vi "musicplayer_next.vi"() -> ()   [LabVIEW 2012]
uses:
  System.Windows.Forms
  <vilib>/Utility/sysdir.llb/System Directory Type.ctl
  NotifyIcon/TypeDefs/NotifyIcon Events.ctl
  NotifyIcon/TypeDefs/NotifyIcon Event Registration Actions.ctl
  musicplayer_glo.vi
  <vilib>/Utility/cursorutil.llb/Set Cursor (Icon Pict).vi
  player_glo.vi
  debug_glo.vi
panel:
  out "ok_str":string
  in  "ok_but":bool
  in  "chase":dbl
  out "playwhile-brake":bool
  out "dataPfad":path
  out "NotifyIcon reference out":refnum<k24>
  out "pause?":bool=TRUE
  out "playlist referenz":refnum<vi>
  out "error-pool":errorcluster caption="Fehler (Ausgang)"
  out "playerkernel referenz":refnum<vi>
  out "version":string
  out "configPfad":path
  in  "ProgressBar":refnum<k24>(container)
  out "verdeckung":bool=TRUE
  in  "switch":bool
  in  "stop":bool
  in  "zufall":bool caption="random"
  out "playalone-titel":string caption="Einzeltitel:"
  in  "nachtitelpausieren":bool caption="last titel"
  in  "wiederholart":enum8{"False", "True", "Mixed"}(c332)
  in  "nechstentitel":bool
  in  "abspielen-einzeln":bool
  in  "pause":bool
  in  "play":bool
  in  "Volume":i64(slide) caption="Lautstärke" min=0 max=100 scale=0.1..100.0
  in  "balance":i8(slide) caption="Balance" scale=-10.0..10.0
  in  "position":ext(slide) caption="Position" scale=-1.0..1.0
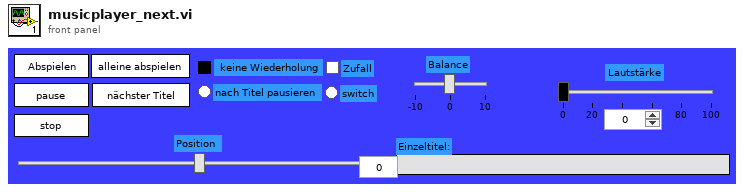
[diagram p1: front panel]
types:
  T1 = typedef "Window Refnum" = refnum<k1>
  T2 = enum32{"Invalid", "Standard", "Closed", "Hidden", "Minimized", "Maximized"}
  T3 = typedef "NotifyIcon Event Registration Actions.ctl" = enum16{"Initial Event Registration", "Add to Event Registration", "Destroy Events and Re-register"}
  T4 = enum8{"Enabled", "Disabled", "Disabled and Grayed Out"}
  T5 = typedef "System Directory Type.ctl" = i32
  T6 = typedef "NotifyIcon Events.ctl" = enum16{"BalloonTipClicked", "BalloonTipClosed", "BalloonTipShown", "Click", "Disposed", "DoubleClick", "MouseClick", "MouseDoubleClick", "MouseDown", "MouseMove", "MouseUp", "MenuItemClick", "MenuItemSelect"}
  T7 = typedef "NotifyIcon Event Data.ctl" = cluster{"NotifyIcon Event":T6, "Data String":string}
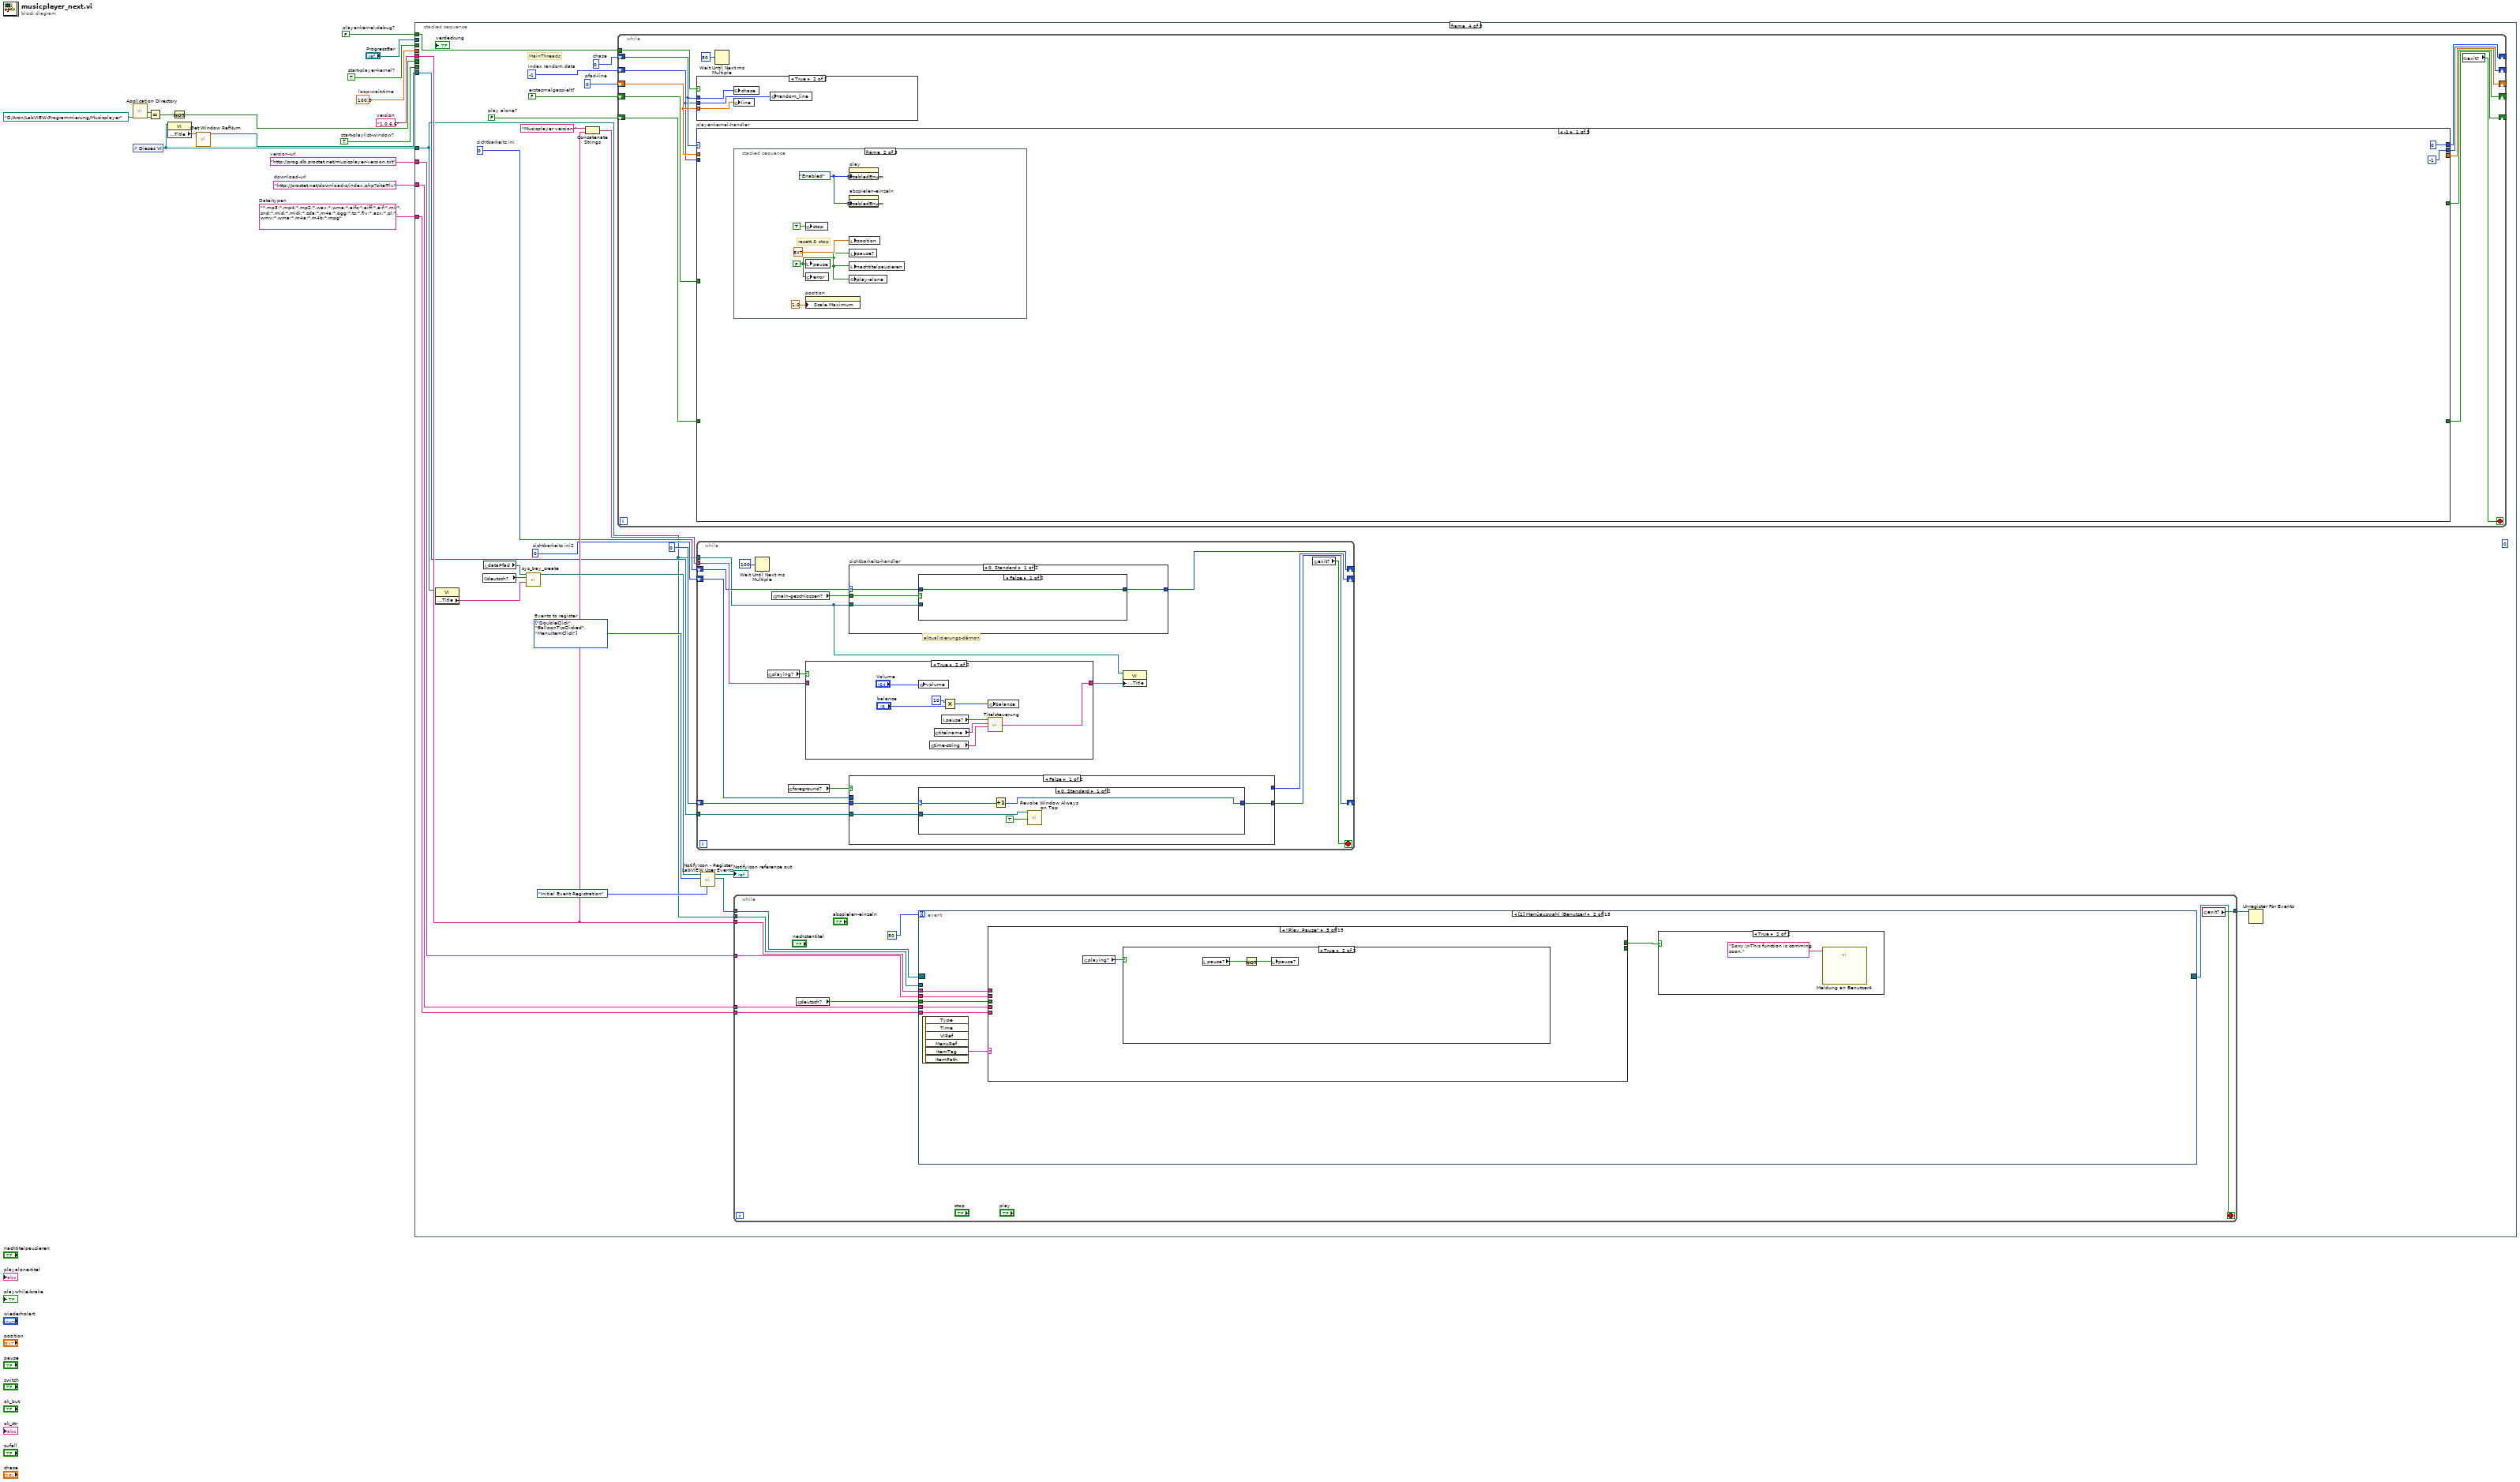
[diagram p0: block diagram]
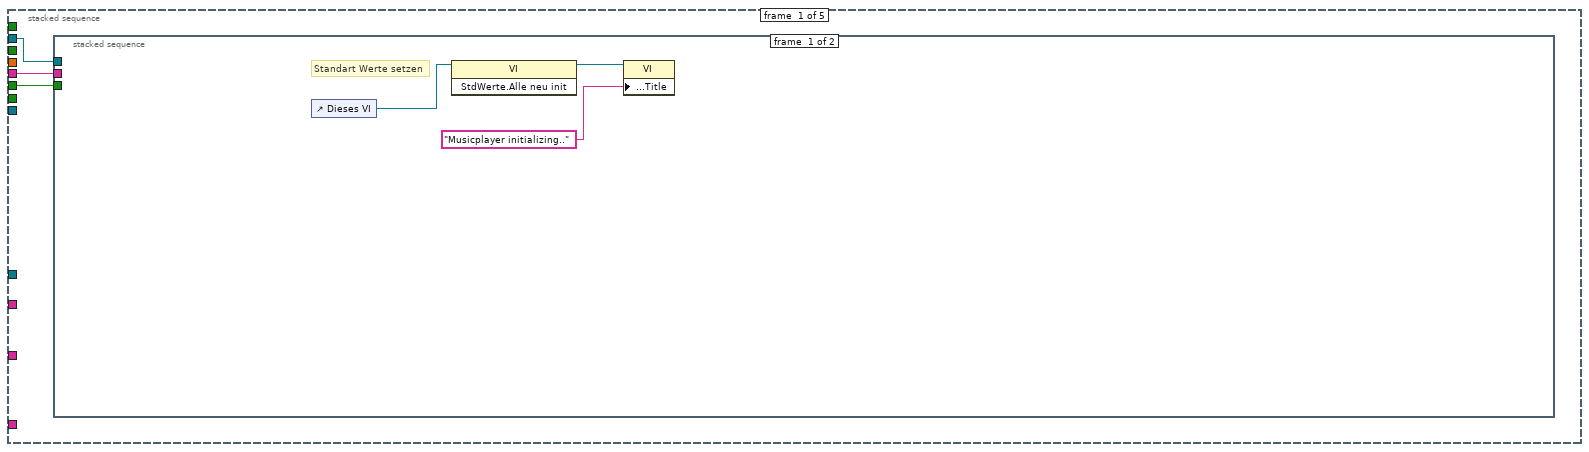
[diagram p2: hidden frame]
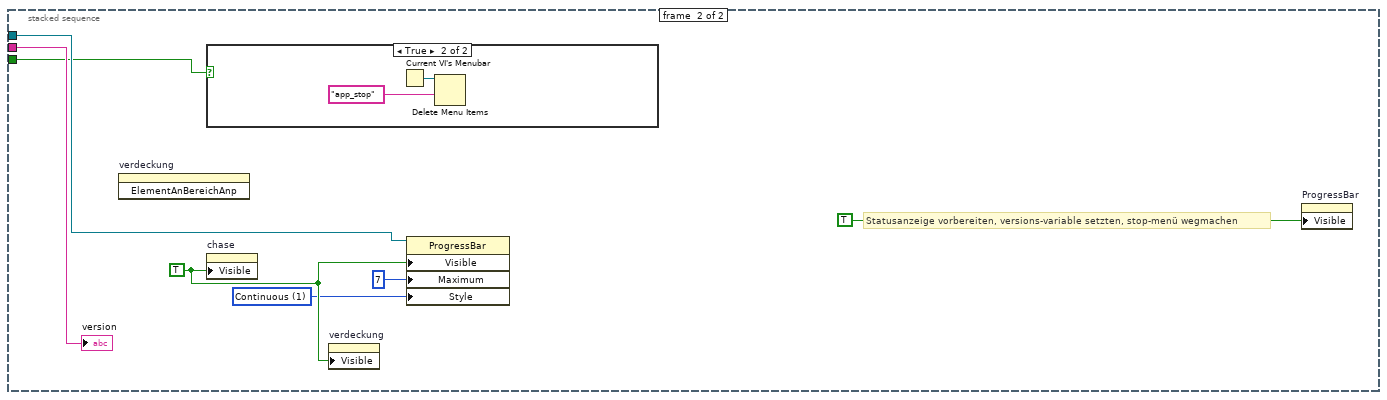
[diagram p3: hidden frame]
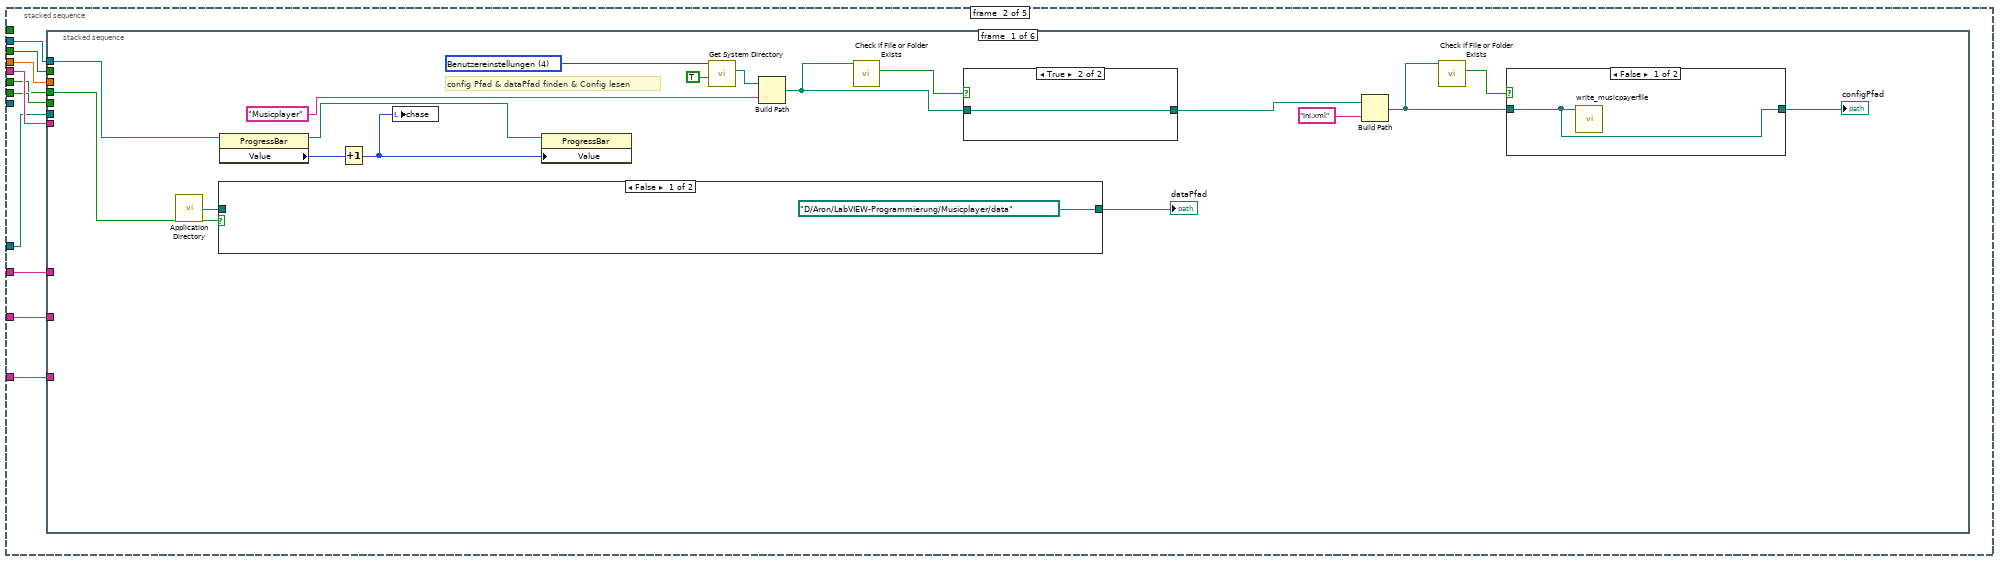
[diagram p5: hidden frame]
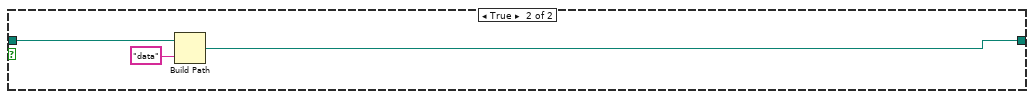
[diagram p6: hidden frame]
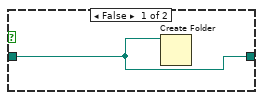
[diagram p8: hidden frame]
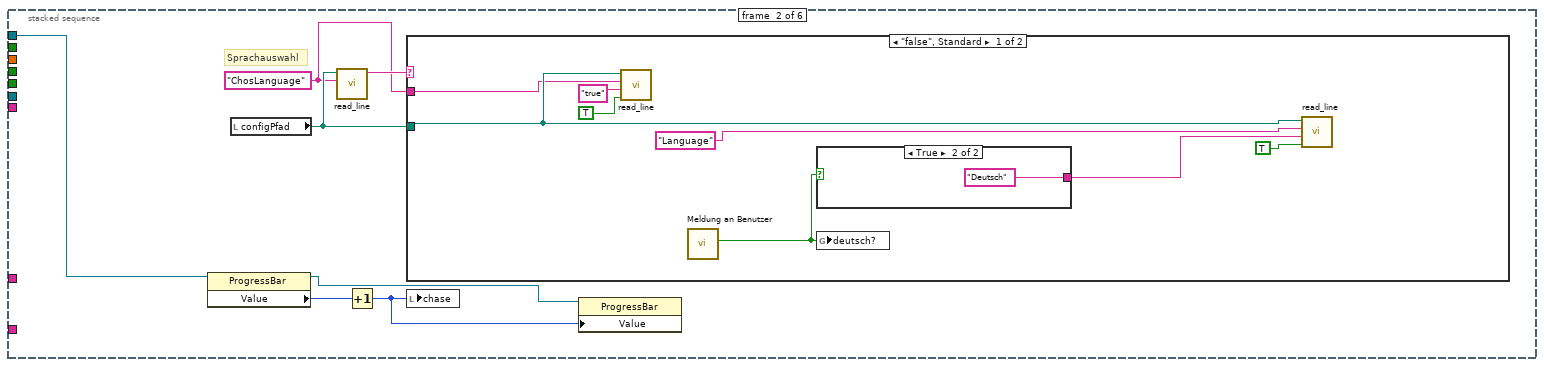
[diagram p9: hidden frame]
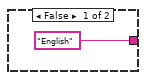
[diagram p10: hidden frame]
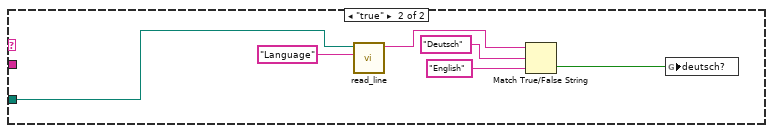
[diagram p11: hidden frame]
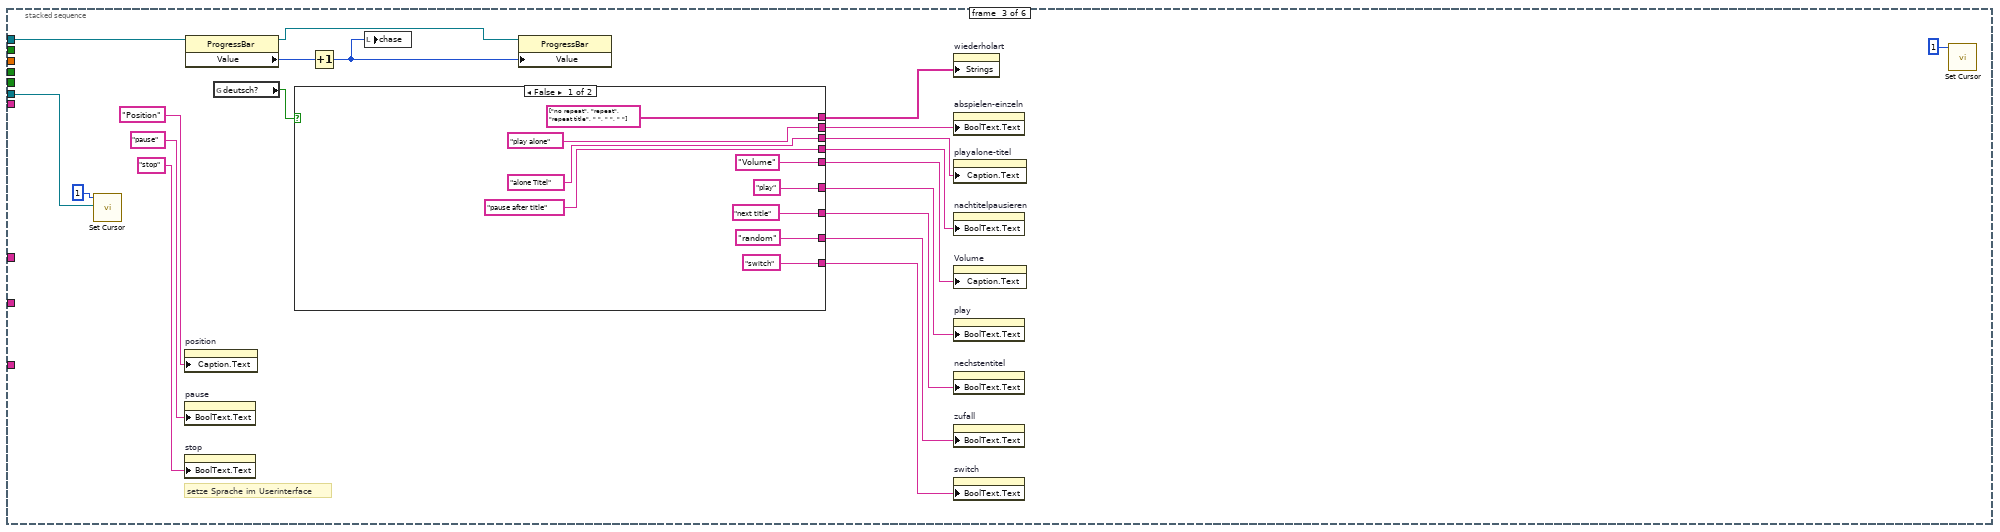
[diagram p12: hidden frame]
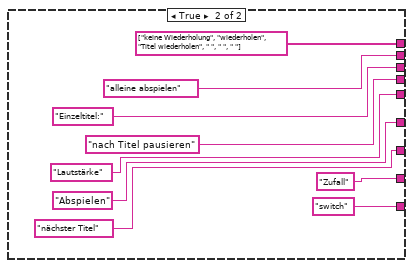
[diagram p13: hidden frame]
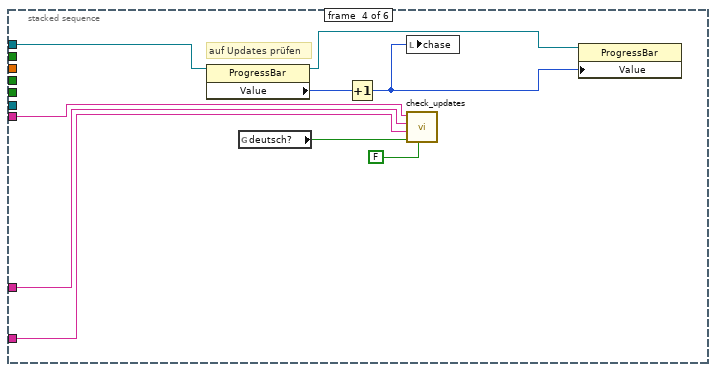
[diagram p14: hidden frame]
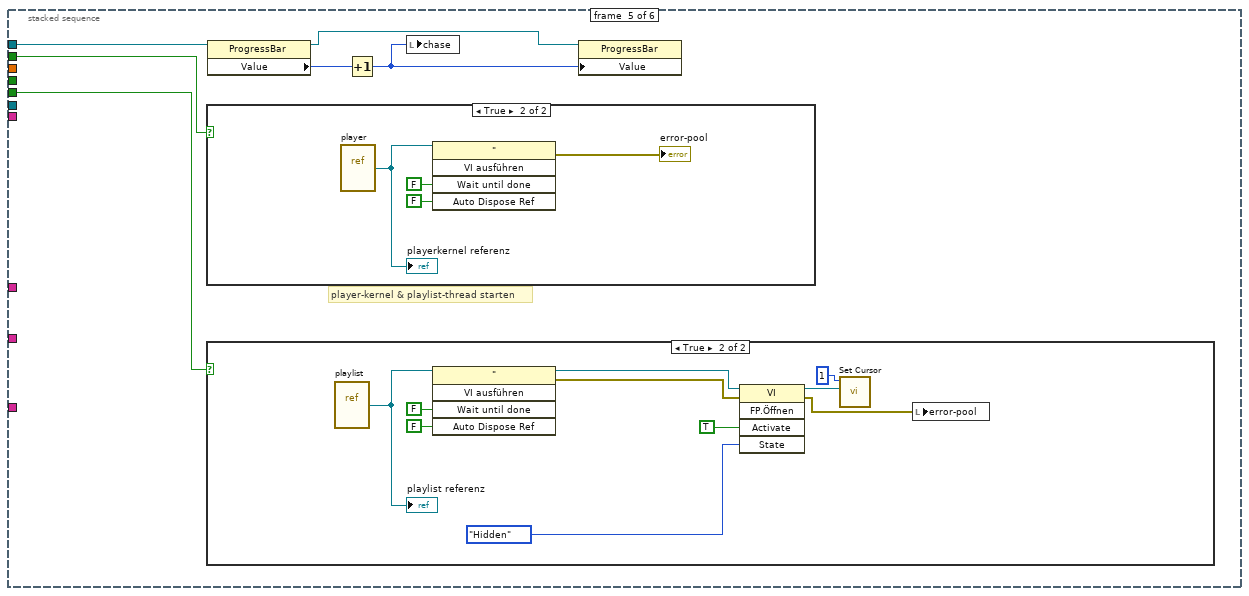
[diagram p15: hidden frame]
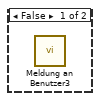
[diagram p16: hidden frame]
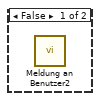
[diagram p17: hidden frame]
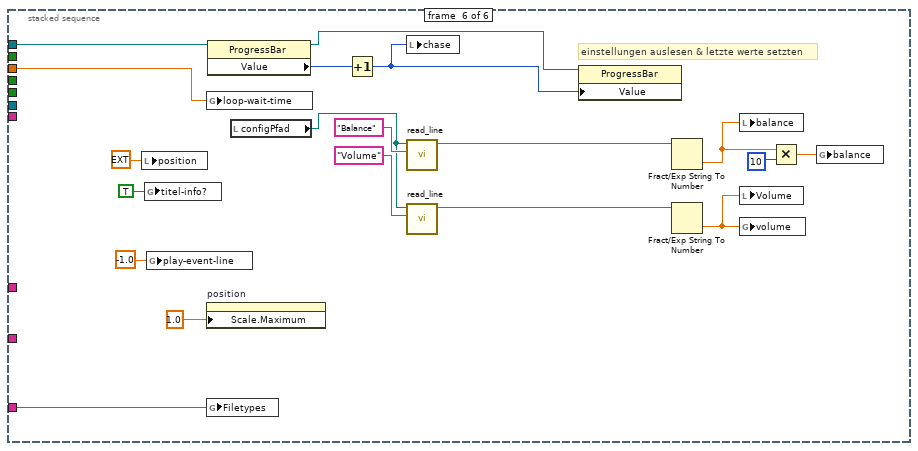
[diagram p18: hidden frame]
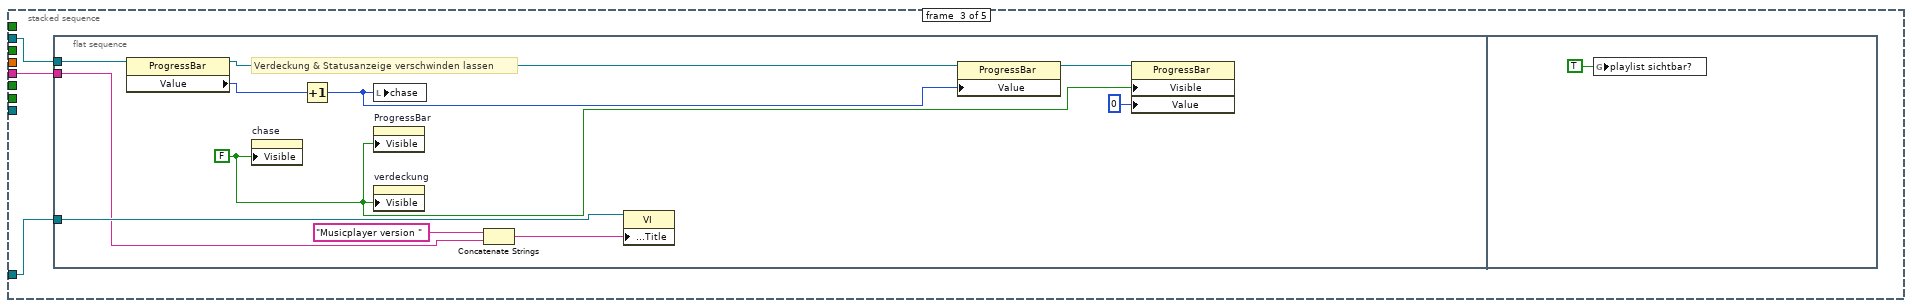
[diagram p19: hidden frame]
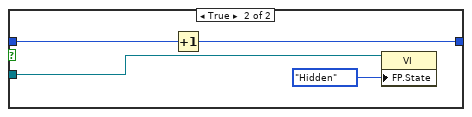
[diagram p20: hidden frame]
diagram:
  w1 = 100.0  # loop-wait-time
  w10 = "*.mp3;*.mp4;*.mp2;*.wav;*.wma;*.aifc;*.aiff;*.aif;*.mi;*.snd;*.mid;*.midi;*.cda;*.m4a;*.ogg;*.ts;*.flv;*.asx;*.pl;*.wmv;*.wma;*.m4a;*.m4b;*.mpg"  # Dateitypen
  w11 = FALSE  # player-kernel-debug?
  w12 = TRUE  # start-playlist-window?
  w13 = TRUE  # start-player-kernel?
  w14 = "http://proctet.net/download-s/index.php?site=lv"  # download-url
  w15 = "http://prog.db.proctet.net/musicplayer-version.txt"  # version-url
  w16 = "1.0.6.6"  # version
  n1 = call <vilib>:"Application Directory.vi"() -> ("Application Directory"=w6:path)
  n2 = control-ref of="Dieses VI"() -> (w4:refnum<vi>)
  n3 = Equal?(x=w6, y=path "D:/Aron/LabVIEW-Programmierung/Musicplayer" ("Zerlegter Pfad")) -> (x = y?=w8:bool)
  n4 = property class="VI"(reference=w4) -> ("Front Panel.Title"=w3:string)  [unwired: 1 in, 2 out]
  n5 = Not(x=w8) -> (.not. x?=w7:bool)
  n6 = call "Get Window RefNum.vi"("window name (\"\")"=w3) -> ("window refnum (NaWR)"=w2:T1)  [unwired: 7 in, 1 out]
  n7 = stacked-sequence {
    tunnel: "ProgressBar" -> [w19 w41 w177 _ _]
    tunnel: w16 -> [w18 w40 w178 w200 _]
    tunnel: w15 -> [_ w39 _ w198 _]
    tunnel: w14 -> [_ w38 _ w199 _]
    tunnel: w13 -> [_ w37 _ _ _]
    tunnel: w12 -> [_ w36 _ _ _]
    tunnel: w4 -> [_ w33 w179 w193 w857]
    tunnel: w11 -> [_ _ _ w212 _]
    tunnel: w10 -> [_ w35 _ w211 _]
    tunnel: w7 -> [w17 w34 _ _ _]
    tunnel: w2 -> [_ _ _ w196 _]
    tunnel: w1 -> [_ w32 _ _ _]
    frame #0 {
      n8 = stacked-sequence {
        tunnel: w19 -> [_ w28]
        tunnel: w18 -> [_ w26]
        tunnel: w17 -> [_ w25]
        frame #0 {
          # "Standart Werte setzen"
          n9 = control-ref of="Dieses VI"() -> (w22:refnum<vi>)
          n10 = invoke class="VI" method="StdWerte.Alle neu init"(reference=w22) -> (reference out=w21:refnum<vi>)  [unwired: 2 in, 2 out]
          n11 = property class="VI"(reference=w21, "Front Panel.Title"="Musicplayer initializing.." ("Frontpanel-Fenster:Titel")) -> ()  [unwired: 1 in, 2 out]
        }
        frame #1 {
          w23 = 1 items=["Blocks", "Continuous", "Marquee"] ("Style")
          w24 = TRUE ("Sichtbar")
          # "Statusanzeige vorbereiten, versions-variable setzten, stop-menü wegmachen"
          n12 = invoke on="verdeckung" class="Bool." method="ElementAnBereichAnp"() -> ()  [unwired: 3 in, 3 out]
          n13 = case shown="True" w25 {
            frame False {
            }
            frame True {
              n14 = Current VI's Menubar() -> (w31:refnum<k9>)
              n15 = Delete Menu Items(7:"app_stop" ("Objekte"), 9:w31) -> ()  [unwired: 2 in, 2 out]
            }
          }
          n16 = property on="chase" class="DigWert (strikt)"("Visible"=w24) -> ()  [unwired: 2 in, 2 out]
          n17 = property on="verdeckung" class="Bool."("Visible"=w24) -> ()  [unwired: 2 in, 2 out]
          n18 = property class="ProgressBar"(reference=w28, "Visible"=w24, "Maximum"=7, "Style"=w23) -> ()  [unwired: 1 in, 2 out]
          n19 = property on="ProgressBar" class="AXCont"("Visible"=TRUE ("Sichtbar")) -> ()  [unwired: 2 in, 2 out]
          "version" <- w26
        }
      }
    }
    frame #1 {
      n20 = stacked-sequence {
        tunnel: w41 -> [w48 w71 w108 w135 w141 w174]
        tunnel: w40 -> [_ _ _ w134 _ _]
        tunnel: w39 -> [_ _ _ w131 _ _]
        tunnel: w38 -> [_ _ _ w130 _ _]
        tunnel: w37 -> [_ _ _ _ w140 _]
        tunnel: w36 -> [_ _ _ _ w139 _]
        tunnel: w35 -> [_ _ _ _ _ w161]
        tunnel: w34 -> [w44 _ _ _ _ _]
        tunnel: w33 -> [_ _ w92 _ _ _]
        tunnel: w32 -> [_ _ _ _ _ w158]
        frame #0 {
          w59 = T5 4 items=["Benutzerverzeichnis"=0, "Benutzer-Desktop"=1, "Benutzerdokumente"=2, "Benutzeranwendungsdaten"=3, "Benutzereinstellungen"=4, "Temporäres Verzeichnis"=5, "Öffentliche Dokumente"=6, "Öffentliche Anwendungsdaten"=7, "Öffentliche Einstellungen"=8, "Öffentlicher Cache"=13, "Systembibliotheken"=9, "Installierte Bibliotheken"=10, "Applikationsdateien"=11, "Boot-Laufwerks-Stammverzeichnis"=12] ("system directory type")
          # "config Pfad & dataPfad finden & Config lesen"
          n21 = call <vilib>:"Application Directory.vi"() -> ("Application Directory"=w43:path)
          n22 = case shown="False" w44 {
            tunnel: w43 -> [_ w63]
            tunnel: [path "D:/Aron/LabVIEW-Programmierung/Musicplayer/data" ("stripped path") w61] -> w45
            frame False {
            }
            frame True {
              n23 = Build Path(base path=w63, name or relative path="data" ("Name oder relativer Pfad")) -> (appended path=w61:path)
            }
          }
          "dataPfad" <- w45
          n24 = property class="ProgressBar"(reference=w48) -> (reference out=w47:refnum<k24>, "Value"=w46:i32)  [unwired: 1 in, 1 out]
          n25 = Increment(x=w46) -> (x+1=w42:i32)
          n26 = local write "chase"(w42) -> ()
          n27 = property class="ProgressBar"(reference=w47, "Value"=w42) -> ()  [unwired: 1 in, 2 out]
          n28 = call <vilib>:"Get System Directory.vi"("create directory if not found? (F)"=TRUE, "system directory type"=w59) -> ("system directory"=w58:path)  [unwired: 9 in]
          n29 = Build Path(base path=w58, name or relative path="Musicplayer" ("Name oder relativer Pfad")) -> (appended path=w54:path)
          n30 = call <vilib>:"Check if File or Folder Exists.vi"("path"=w54) -> ("file or folder exists?"=w55:bool)  [unwired: 8 in, 2 out]
          n31 = case shown="True" w55 {
            tunnel: w54 -> [w66 w67]
            tunnel: [w66 w67] -> w53
            frame False {
              n32 = Create Folder(path (use dialog)=w66) -> ()  [unwired: 2 in, 3 out]
            }
            frame True {
            }
          }
          n33 = Build Path(base path=w53, name or relative path="ini.xml" ("Name oder relativer Pfad")) -> (appended path=w50:path)
          n34 = call <vilib>:"Check if File or Folder Exists.vi"("path"=w50) -> ("file or folder exists?"=w51:bool)  [unwired: 8 in, 2 out]
          n35 = case shown="False" w51 {
            tunnel: w50 -> [w64 w65]
            tunnel: [w64 w65] -> w49
            frame False {
              n36 = call "write_musicpayerfile.vi"("New XML File path"=w64) -> ()  [unwired: 10 in, 1 out]
            }
            frame True {
            }
          }
          "configPfad" <- w49
        }
        frame #1 {
          w68 = "ChosLanguage" ("Search objekt")
          # "Sprachauswahl"
          n37 = property class="ProgressBar"(reference=w71) -> (reference out=w73:refnum<k24>, "Value"=w72:i32)  [unwired: 1 in, 1 out]
          n38 = local read "configPfad"() -> (w70:path)
          n39 = call "read_line.vi"("Search objekt"=w68, "path to XML document"=w70) -> ("Value"=w74:string)  [unwired: 9 in]
          n40 = Increment(x=w72) -> (x+1=w69:i32)
          n41 = case shown="\"false\", Standard" w74 {
            tunnel: w70 -> [w78 w89]
            tunnel: w68 -> [w75 _]
            frame "false", Default {
              n42 = call "read_line.vi"("write"=TRUE, "Writedata"="true", "Search objekt"=w75, "path to XML document"=w78) -> ()  [unwired: 7 in, 1 out]
              n43 = call "Meldung an Benutzer"() -> ("German"=w82:bool)  [unwired: 10 in, 1 out]
              n44 = case shown="True" w82 {
                tunnel: ["English" "Deutsch"] -> w76
                frame False {
                }
                frame True {
                }
              }
              n45 = global write "musicplayer_glo.vi" "deutsch?"(w82) -> ()
              n46 = call "read_line.vi"("write"=TRUE, "Writedata"=w76, "Search objekt"="Language", "path to XML document"=w78) -> ()  [unwired: 7 in, 1 out]
            }
            frame "true" {
              n47 = call "read_line.vi"("Search objekt"="Language", "path to XML document"=w89) -> ("Value"=w88:string)  [unwired: 9 in]
              n48 = Match True/False String(2:"English" ("False-String"), 3:"Deutsch" ("True-String"), 4:w88) -> (0:w85:bool)  [unwired: 1 out]
              n49 = global write "musicplayer_glo.vi" "deutsch?"(w85) -> ()
            }
          }
          n50 = local write "chase"(w69) -> ()
          n51 = property class="ProgressBar"(reference=w73, "Value"=w69) -> ()  [unwired: 1 in, 2 out]
        }
        frame #2 {
          # "setze Sprache im Userinterface"
          n52 = call-poly <vilib>:"Set Cursor.vi"("VI reference (current VI)"=w92, "icon"=u16 1) -> ()  [unwired: 8 in, 2 out]
          n53 = property on="position" class="Schieber (strikt)"("Caption.Text"="Position") -> ()  [unwired: 2 in, 2 out]
          n54 = property on="pause" class="Bool. (strikt)"("BoolText.Text"="pause") -> ()  [unwired: 2 in, 2 out]
          n55 = property on="stop" class="Bool."("BoolText.Text"="stop") -> ()  [unwired: 2 in, 2 out]
          n56 = property class="ProgressBar"(reference=w108) -> (reference out=w110:refnum<k24>, "Value"=w109:i32)  [unwired: 1 in, 1 out]
          n57 = global read "musicplayer_glo.vi" "deutsch?"() -> (w107:bool)
          n58 = case shown="False" w107 {
            tunnel: [string[] ["no repeat", "repeat", "repeat title", " ", " ", " "] string[] ["keine Wiederholung", "wiederholen", "Titel wiederholen", " ", " ", " "]] -> w100
            tunnel: ["play" "Abspielen"] -> w106
            tunnel: ["play alone" "alleine abspielen"] -> w105
            tunnel: ["next title" "nächster Titel"] -> w103
            tunnel: ["pause after title" "nach Titel pausieren"] -> w101
            tunnel: ["random" "Zufall"] -> w99
            tunnel: ["switch" "switch"] -> w98
            tunnel: ["Volume" "Lautstärke"] -> w97
            tunnel: ["alone Titel" "Einzeltitel:"] -> w95
            frame False {
            }
            frame True {
            }
          }
          n59 = Increment(x=w109) -> (x+1=w94:i32)
          n60 = local write "chase"(w94) -> ()
          n61 = property class="ProgressBar"(reference=w110, "Value"=w94) -> ()  [unwired: 1 in, 2 out]
          n62 = property on="wiederholart" class="3ZustandsFeld (strikt)"("Strings"=w100) -> ()  [unwired: 2 in, 2 out]
          n63 = property on="abspielen-einzeln" class="Bool."("BoolText.Text"=w105) -> ()  [unwired: 2 in, 2 out]
          n64 = property on="playalone-titel" class="Str"("Caption.Text"=w95) -> ()  [unwired: 2 in, 2 out]
          n65 = property on="nachtitelpausieren" class="Bool. (strikt)"("BoolText.Text"=w101) -> ()  [unwired: 2 in, 2 out]
          n66 = property on="Volume" class="Schieber (strikt)"("Caption.Text"=w97) -> ()  [unwired: 2 in, 2 out]
          n67 = property on="play" class="Bool."("BoolText.Text"=w106) -> ()  [unwired: 2 in, 2 out]
          n68 = property on="nechstentitel" class="Bool."("BoolText.Text"=w103) -> ()  [unwired: 2 in, 2 out]
          n69 = property on="zufall" class="Bool. (strikt)"("BoolText.Text"=w99) -> ()  [unwired: 2 in, 2 out]
          n70 = property on="switch" class="Bool. (strikt)"("BoolText.Text"=w98) -> ()  [unwired: 2 in, 2 out]
          n71 = call-poly <vilib>:"Set Cursor.vi"("icon"=u16 1) -> ()  [unwired: 9 in, 2 out]
        }
        frame #3 {
          # "auf Updates prüfen"
          n72 = property class="ProgressBar"(reference=w135) -> (reference out=w137:refnum<k24>, "Value"=w136:i32)  [unwired: 1 in, 1 out]
          n73 = global read "musicplayer_glo.vi" "deutsch?"() -> (w133:bool)
          n74 = Increment(x=w136) -> (x+1=w129:i32)
          n75 = local write "chase"(w129) -> ()
          n76 = call "check_updates.vi"("dialog by newest version?"=FALSE, "german?"=w133, "downloadpath"=w130, "get-path"=w131, "current version"=w134) -> ()  [unwired: 6 in, 1 out]
          n77 = property class="ProgressBar"(reference=w137, "Value"=w129) -> ()  [unwired: 1 in, 2 out]
        }
        frame #4 {
          # "player-kernel & playlist-thread starten"
          n78 = case shown="True" w140 {
            frame False {
              n79 = call "Meldung an Benutzer2"() -> ()  [unwired: 10 in, 2 out]
            }
            frame True {
              n80 = vi-ref "player.vi"() -> (w155:refnum<vi>)
              "playerkernel referenz" <- w155
              n81 = invoke class="\"" method="VI ausführen"(reference=w155, "Wait until done"=FALSE ("Warten bis beendet"), "Auto Dispose Ref"=FALSE ("Referenz automatisch schließen")) -> (error out=→"error-pool":errorcluster)  [unwired: 2 in, 4 out]
            }
          }
          n82 = case shown="True" w139 {
            frame False {
              n83 = call "Meldung an Benutzer3"() -> ()  [unwired: 10 in, 2 out]
            }
            frame True {
              n84 = vi-ref "playlist.vi"() -> (w151:refnum<vi>)
              "playlist referenz" <- w151
              n85 = invoke class="\"" method="VI ausführen"(reference=w151, "Wait until done"=FALSE ("Warten bis beendet"), "Auto Dispose Ref"=FALSE ("Referenz automatisch schließen")) -> (reference out=w150:refnum<vi>, error out=w149:errorcluster)  [unwired: 2 in, 3 out]
              n86 = invoke class="VI" method="FP.Öffnen"(reference=w150, error in=w149, "Activate"=TRUE ("Aktivieren?"), "State"=T2."Hidden" ("Zustand")) -> (reference out=w144:refnum<vi>, error out=w148:errorcluster)  [unwired: 1 in, 3 out]
              n87 = call-poly <vilib>:"Set Cursor.vi"("VI reference (current VI)"=w144, "icon"=u16 1) -> ()  [unwired: 8 in, 2 out]
              n88 = local write "error-pool"(w148) -> ()
            }
          }
          n89 = property class="ProgressBar"(reference=w141) -> (reference out=w143:refnum<k24>, "Value"=w142:i32)  [unwired: 1 in, 1 out]
          n90 = Increment(x=w142) -> (x+1=w138:i32)
          n91 = local write "chase"(w138) -> ()
          n92 = property class="ProgressBar"(reference=w143, "Value"=w138) -> ()  [unwired: 1 in, 2 out]
        }
        frame #5 {
          # "einstellungen auslesen & letzte werte setzten"
          n93 = local write "position"(ext 1.0 ("position")) -> ()
          n94 = global write "musicplayer_glo.vi" "titel-info?"(TRUE ("titel-info?")) -> ()
          n95 = global write "musicplayer_glo.vi" "play-event-line"(-1.0 ("play-event-line")) -> ()
          n96 = global write "player_glo.vi" "loop-wait-time"(w158) -> ()
          n97 = property on="position" class="Schieber (strikt)"("Scale.Maximum"=1.0 ("Skalierung.Bereich:Maximum")) -> ()  [unwired: 2 in, 2 out]
          n98 = global write "musicplayer_glo.vi" "Filetypes"(w161) -> ()
          n99 = property class="ProgressBar"(reference=w174) -> (reference out=w176:refnum<k24>, "Value"=w175:i32)  [unwired: 1 in, 1 out]
          n100 = local read "configPfad"() -> (w167:path)
          n101 = Increment(x=w175) -> (x+1=w159:i32)
          n102 = local write "chase"(w159) -> ()
          n103 = call "read_line.vi"("Search objekt"="Balance", "path to XML document"=w167) -> ("Value"=w172:string)  [unwired: 9 in]
          n104 = call "read_line.vi"("Search objekt"="Volume", "path to XML document"=w167) -> ("Value"=w168:string)  [unwired: 9 in]
          n105 = property class="ProgressBar"(reference=w176, "Value"=w159) -> ()  [unwired: 1 in, 2 out]
          n106 = Fract/Exp String To Number(string=w172) -> (number=w165:dbl)  [unwired: 4 out]
          n107 = Fract/Exp String To Number(string=w168) -> (number=w166:dbl)  [unwired: 4 out]
          n108 = local write "balance"(w165) -> ()
          n109 = local write "Volume"(w166) -> ()
          n110 = global write "player_glo.vi" "volume"(w166) -> ()
          n111 = Multiply(x=w165, y=10 ("Offset nach Zahl")) -> (x*y=w170:dbl)
          n112 = global write "player_glo.vi" "balance"(w170) -> ()
        }
      }
    }
    frame #2 {
      n113 = flat-sequence {
        tunnel: w179 -> [w189]
        tunnel: w178 -> [w186]
        tunnel: w177 -> [w183]
        frame #0 {
          w180 = FALSE ("Visible")
          # "Verdeckung & Statusanzeige verschwinden lassen"
          n114 = property class="ProgressBar"(reference=w183) -> (reference out=w185:refnum<k24>, "Value"=w184:i32)  [unwired: 1 in, 1 out]
          n115 = property on="chase" class="DigWert (strikt)"("Visible"=w180) -> ()  [unwired: 2 in, 2 out]
          n116 = Increment(x=w184) -> (x+1=w181:i32)
          n117 = local write "chase"(w181) -> ()
          n118 = property on="ProgressBar" class="AXCont"("Visible"=w180) -> ()  [unwired: 2 in, 2 out]
          n119 = property on="verdeckung" class="Bool."("Visible"=w180) -> ()  [unwired: 2 in, 2 out]
          n120 = Concatenate Strings("Musicplayer version " ("String"), w186) -> (w188:string)
          n121 = property class="VI"(reference=w189, "Front Panel.Title"=w188) -> ()  [unwired: 1 in, 2 out]
          n122 = property class="ProgressBar"(reference=w185, "Value"=w181) -> (reference out=w182:refnum<k24>)  [unwired: 1 in, 1 out]
          n123 = property class="ProgressBar"(reference=w182, "Visible"=w180, "Value"=0) -> ()  [unwired: 1 in, 2 out]
        }
        frame #1 {
          n124 = global write "musicplayer_glo.vi" "playlist sichtbar?"(TRUE ("playlist sichtbar?")) -> ()
        }
      }
    }
    frame #3 {
      w195 = 0  # sichtbarkeits ini2
      w197 = 0  # sichtbarkeits ini
      w206 = T6[] [enum."DoubleClick", enum."BalloonTipClicked", enum."MenuItemClick"] items=["BalloonTipClicked", "BalloonTipClosed", "BalloonTipShown", "Click", "Disposed", "DoubleClick", "MouseClick", "MouseDoubleClick", "MouseDown", "MouseMove", "MouseUp", "MenuItemClick", "MenuItemSelect"]  # Events to register
      (unwired) 0
      w213 = -1  # index random data
      w214 = FALSE  # play alone?
      w215 = 0  # pfad-line
      w216 = FALSE  # erstesmalgespielt?
      w217 = 0  # chase
      # "MainThreads"
      n125 = property class="VI"(reference=w193) -> ("Front Panel.Title"=w192:string)  [unwired: 1 in, 2 out]
      n126 = global read "musicplayer_glo.vi" "deutsch?"() -> (w203:bool)
      n127 = local read "dataPfad"() -> (w201:path)
      n128 = call "sys_tray_create.vi"("hover-text"=w192, "deutsch?"=w203, "data_pfad"=w201) -> ("NotifyIcon reference out"=w207:refnum<k24>)  [unwired: 8 in]
      n129 = Concatenate Strings("Musicplayer version " ("String"), w200) -> (w209:string)
      n130 = while {
        shift-right: [w495] -> _
        shift-left: w217 -> [w486]
        shift-right: [w494] -> _
        shift-left: w215 -> [w485]
        shift-right: [w493] -> _
        shift-left: w214 -> [w492]
        shift-right: [w490] -> _
        shift-left: w216 -> [w491]
        shift-right: [w489] -> _
        shift-left: w213 -> [w484]
        tunnel: w212 -> [w488]
        stop <- w487 stop-if-true
        n131 = case shown="True" w488 {
          tunnel: w486 -> [_ w499]
          tunnel: w485 -> [_ w498]
          tunnel: w484 -> [_ w497]
          frame False {
          }
          frame True {
            n132 = global write "debug_glo.vi" "chase"(w499) -> ()
            n133 = global write "debug_glo.vi" "line"(w498) -> ()
            n134 = global write "debug_glo.vi" "random_line"(w497) -> ()
          }
        }
        n135 = case "player-kernel-handler" shown="-1" w486 {
          selector: w486 -> [_ w511 w530 _ _]
          tunnel: [0 w510 w528 w729 w772] -> w495
          tunnel: [_ -1 w525 w733 w773] -> w494
          tunnel: w485 -> [_ _ w526 w733 w773]
          tunnel: [_ _ w531 w732 w769] -> w493
          tunnel: w492 -> [_ _ _ w732 w769]
          tunnel: w491 -> [_ _ w527 w731 _]
          tunnel: [_ _ _ w731 w770] -> w490
          tunnel: w484 -> [_ _ w524 w730 w771]
          tunnel: [-1 -1 w522 w730 w771] -> w489
          frame -1 {
            n136 = stacked-sequence {
              frame #0 {
                n137 = global write "musicplayer_glo.vi" "stop-event"(TRUE ("stop-event")) -> ()
              }
              frame #1 {
                w507 = T4."Enabled" ("Deaktiviert")
                w504 = FALSE ("play-alone")
                # "resett & stop"
                n138 = global write "player_glo.vi" "stop"(TRUE ("stop")) -> ()
                n139 = local write "pause"(w504) -> ()
                n140 = global write "player_glo.vi" "error"(w504) -> ()
                n141 = property on="position" class="Schieber (strikt)"("Scale.Maximum"=1.0 ("Skalierung.Bereich:Maximum")) -> ()  [unwired: 2 in, 2 out]
                n142 = property on="play" class="Bool."("DisabledEnum"=w507) -> ()  [unwired: 2 in, 2 out]
                n143 = property on="abspielen-einzeln" class="Bool."("DisabledEnum"=w507) -> ()  [unwired: 2 in, 2 out]
                n144 = local write "position"(ext 0.0 ("position")) -> ()
                n145 = local write "pause?"(w504) -> ()
                n146 = local write "nachtitelpausieren"(w504) -> ()
                n147 = global write "musicplayer_glo.vi" "play-alone"(w504) -> ()
              }
              frame #2 {
                n148 = global write "musicplayer_glo.vi" "stop-event"(FALSE ("stop-event")) -> ()
              }
            }
          }
          frame 0, Default {
            n149 = global read "musicplayer_glo.vi" "play-event"() -> (w512:bool)
            n150 = case "play-event-handler" shown="True" w512 {
              tunnel: w511 -> [w514 _]
              tunnel: [w514 1] -> w510
              frame False {
              }
              frame True {
              }
            }
          }
          frame 1 {
            w518 = FALSE ("stop-event")
            w521 = T4."Disabled and Grayed Out" ("Deaktiviert")
            n151 = global read "musicplayer_glo.vi" "play-alone"() -> (w531:bool)
            n152 = global read "musicplayer_glo.vi" "play-event"() -> (w534:bool)
            n153 = local write "pause"(w518) -> ()
            n154 = local read "nachtitelpausieren"() -> (w517:bool)
            n155 = global read "musicplayer_glo.vi" "play-event-line"() -> (w532:dbl)
            n156 = global write "musicplayer_glo.vi" "stop-event"(w518) -> ()
            n157 = local write "playwhile-brake"(w518) -> ()
            n158 = local write "pause?"(w518) -> ()
            n159 = case shown="True" w517 {
              frame False {
              }
              frame True {
                n160 = property on="nachtitelpausieren" class="Bool. (strikt)"("DisabledEnum"=T4."Disabled and Grayed Out" ("Deaktiviert")) -> ()  [unwired: 2 in, 2 out]
              }
            }
            n161 = local read "switch"() -> (w519:bool)
            n162 = local read "zufall"() -> (w523:bool)
            n163 = property on="play" class="Bool."("DisabledEnum"=w521) -> ()  [unwired: 2 in, 2 out]
            n164 = property on="abspielen-einzeln" class="Bool."("DisabledEnum"=w521) -> ()  [unwired: 2 in, 2 out]
            n165 = case "play-event?" shown="False" w534 {
              tunnel: w531 -> [w548 w703]
              tunnel: w532 -> [_ w697]
              tunnel: [w547 w702] -> w533
              tunnel: [w546 _] -> w529
              tunnel: w527 -> [w545 _]
              tunnel: w526 -> [w544 _]
              tunnel: [w543 w701] -> w525
              tunnel: w524 -> [w541 w700]
              tunnel: w523 -> [w542 w699]
              tunnel: [w540 w698] -> w522
              tunnel: [_ FALSE ("play-event")] -> w520
              tunnel: w519 -> [w539 _]
              frame False {
                n166 = case "switch?" shown="False" w539 {
                  tunnel: w548 -> [w557 w663]
                  tunnel: [w556 w658] -> w547
                  tunnel: [w555 w661] -> w546
                  tunnel: w545 -> [w554 _]
                  tunnel: w544 -> [w553 _]
                  tunnel: [w549 w659] -> w543
                  tunnel: w542 -> [w552 w662]
                  tunnel: w541 -> [w551 _]
                  tunnel: [w550 w660] -> w540
                  frame False {
                    n167 = local read "wiederholart"() -> (w558:enum8{"False", "True", "Mixed"})
                    n168 = case "play-alone?" shown="False" w557 {
                      tunnel: w558 -> [w565 w648]
                      tunnel: [w562 w647] -> w556
                      tunnel: [w561 w646] -> w555
                      tunnel: w554 -> [_ w645]
                      tunnel: w553 -> [w566 w643]
                      tunnel: w552 -> [w563 _]
                      tunnel: w551 -> [w564 _]
                      tunnel: [w559 -1] -> w550
                      tunnel: [w560 w643] -> w549
                      frame False {
                        n169 = case "zufall?" shown="False" w563 {
                          tunnel: w565 -> [w568 w602]
                          tunnel: [w572 w599] -> w562
                          tunnel: [w571 w601] -> w561
                          tunnel: [w570 w595] -> w560
                          tunnel: w564 -> [_ w597]
                          tunnel: [-1 w600] -> w559
                          tunnel: w566 -> [w567 _]
                          frame False {
                            n170 = global read "musicplayer_glo.vi" "pfade"() -> (w577:string[])
                            n171 = Array Size(array=w577) -> (size(s)=w576:i32)
                            n172 = Subtract(x=w576, y=1 ("Größe(n)")) -> (x-y=w574:i32)
                            n173 = Equal?(x=w567, y=w574) -> (x = y?=w573:bool)
                            n174 = case "lezter titel?" shown="True" w573 {
                              tunnel: w568 -> [w579 w591]
                              tunnel: [w581 w589] -> w572
                              tunnel: [_ w592] -> w571
                              tunnel: [w580 w588] -> w570
                              tunnel: w567 -> [w578 _]
                              frame False {
                                n175 = Equal?(x=w579, y=enum8{"False", "True", "Mixed"}."Mixed") -> (x = y?=w582:bool)
                                n176 = case "titel wiederholen?" shown="False" w582 {
                                tunnel: [w586 w587] -> w580
                                tunnel: w578 -> [w585 w587]
                                frame False {
                                n177 = Increment(x=w585) -> (x+1=w586:ext)
                                }
                                frame True {
                                }
                                }
                                n178 = global read "musicplayer_glo.vi" "pfade"() -> (w583:string[])
                                n179 = Index Array(array=w583, index=w580) -> (element=w581:string)
                              }
                              frame True {
                                n180 = case "wiederholart" shown="\"False\", Standard" w591 {
                                tunnel: [TRUE _ _] -> w592
                                tunnel: [_ 0 _] -> w588
                                frame "False", Default {
                                }
                                frame "True" {
                                }
                                frame "Mixed" {
                                }
                                }
                                n181 = global read "musicplayer_glo.vi" "pfade"() -> (w590:string[])
                                n182 = Index Array(array=w590, index=w588) -> (element=w589:string)
                              }
                            }
                          }
                          frame True {
                            n183 = Not Equal?(x=w597, y=-1) -> (x != y?=w596:bool)
                            n184 = case "zufallswerte generiert?" shown="False" w596 {
                              tunnel: w602 -> [_ w618]
                              tunnel: [_ w617] -> w601
                              tunnel: [w605 w616] -> w600
                              tunnel: w597 -> [_ w614]
                              tunnel: [w604 w615] -> w599
                              tunnel: [w603 w612] -> w595
                              frame False {
                                n185 = stacked-sequence {
                                tunnel: [_ w609] -> w605
                                tunnel: [_ w608] -> w604
                                tunnel: [_ w606] -> w603
                                frame #0 {
                                n186 = call "write_random_data.vi"() -> ()  [unwired: 12 in]
                                }
                                frame #1 {
                                w609 = 0
                                n187 = global read "musicplayer_glo.vi" "random-data"() -> (w607:ext[])
                                n188 = Index Array(array=w607, index=w609) -> (element=w606:ext)
                                n189 = global read "musicplayer_glo.vi" "pfade"() -> (w610:string[])
                                n190 = Index Array(array=w610, index=w606) -> (element=w608:string)
                                }
                                }
                              }
                              frame True {
                                n191 = global read "musicplayer_glo.vi" "random-data"() -> (w611:ext[])
                                n192 = Array Size(array=w611) -> (size(s)=w613:i32)
                                n193 = Greater Or Equal?(x=w614, y=w613) -> (x >= y?=w619:bool)
                                n194 = case "lezter zufallswert?" shown="True" w619 {
                                tunnel: w618 -> [w624 w639]
                                tunnel: [_ w638] -> w617
                                tunnel: [w622 w634] -> w616
                                tunnel: w614 -> [w623 w637]
                                tunnel: [w627 w635] -> w615
                                tunnel: w611 -> [w621 w633]
                                tunnel: [w620 w632] -> w612
                                frame False {
                                n195 = Equal?(x=w624, y=enum8{"False", "True", "Mixed"}."Mixed") -> (x = y?=w625:bool)
                                n196 = case "titel wiederholen?" shown="True" w625 {
                                tunnel: w623 -> [w629 w631]
                                tunnel: [w630 w631] -> w622
                                frame False {
                                n197 = Increment(x=w629) -> (x+1=w630:i32)
                                }
                                frame True {
                                }
                                }
                                n198 = Index Array(array=w621, index=w622) -> (element=w620:ext)
                                n199 = global read "musicplayer_glo.vi" "pfade"() -> (w628:string[])
                                n200 = Index Array(array=w628, index=w620) -> (element=w627:string)
                                }
                                frame True {
                                n201 = case "wiederholung?" shown="\"Mixed\"" w639 {
                                tunnel: [TRUE _ _] -> w638
                                tunnel: [_ 0 w642] -> w634
                                tunnel: w637 -> [_ _ w642]
                                frame "False", Default {
                                }
                                frame "True" {
                                }
                                frame "Mixed" {
                                }
                                }
                                n202 = Index Array(array=w633, index=w634) -> (element=w632:ext)
                                n203 = global read "musicplayer_glo.vi" "pfade"() -> (w636:string[])
                                n204 = Index Array(array=w636, index=w632) -> (element=w635:string)
                                }
                                }
                              }
                            }
                          }
                        }
                      }
                      frame True {
                        n205 = case "wiederholgung?" shown="\"False\", Standard" w648 {
                          tunnel: [w649 w654 w655] -> w647
                          tunnel: [w651 _ _] -> w646
                          tunnel: w645 -> [w650 _ _]
                          frame "False", Default {
                            n206 = case "schonmal gespielt?" shown="True" w650 {
                              tunnel: [_ TRUE] -> w651
                              tunnel: [w652 _] -> w649
                              frame False {
                                n207 = global read "musicplayer_glo.vi" "playlone-lied-Pfad"() -> (w652:string)
                              }
                              frame True {
                              }
                            }
                          }
                          frame "True" {
                            n208 = global read "musicplayer_glo.vi" "playlone-lied-Pfad"() -> (w654:string)
                          }
                          frame "Mixed" {
                            n209 = global read "musicplayer_glo.vi" "playlone-lied-Pfad"() -> (w655:string)
                          }
                        }
                      }
                    }
                  }
                  frame True {
                    n210 = case "play-alone?" shown="True" w663 {
                      tunnel: w662 -> [_ w677]
                      tunnel: [_ w672] -> w661
                      tunnel: [-1 w671] -> w660
                      tunnel: [_ w669] -> w659
                      tunnel: [w665 w668] -> w658
                      tunnel: [TRUE FALSE] -> w657
                      frame False {
                        n211 = global read "musicplayer_glo.vi" "playlone-lied-Pfad"() -> (w665:string)
                      }
                      frame True {
                        n212 = global read "musicplayer_glo.vi" "pfade"() -> (w675:string[])
                        n213 = Index Array(array=w675, index=0 ("Index")) -> (element=w670:string)
                        n214 = Not Equal?(x=w670, y="") -> (x != y?=w673:bool)
                        n215 = case "leere playlist?" shown="True" w673 {
                          tunnel: w677 -> [_ w684]
                          tunnel: [TRUE _] -> w672
                          tunnel: [-1 w682] -> w671
                          tunnel: w670 -> [_ w683]
                          tunnel: [_ w681] -> w669
                          tunnel: [_ w680] -> w668
                          frame False {
                          }
                          frame True {
                            n216 = case "zufall?" shown="True" w684 {
                              tunnel: w683 -> [w685 _]
                              tunnel: [-1 w690] -> w682
                              tunnel: [0 w688] -> w681
                              tunnel: [w685 w689] -> w680
                              frame False {
                              }
                              frame True {
                                n217 = stacked-sequence {
                                tunnel: [_ w693] -> _
                                tunnel: [_ w694] -> w689
                                tunnel: [_ w693] -> w690
                                tunnel: [_ w691] -> w688
                                frame #0 {
                                n218 = call "write_random_data.vi"() -> ()  [unwired: 12 in]
                                }
                                frame #1 {
                                w693 = 0
                                n219 = global read "musicplayer_glo.vi" "random-data"() -> (w692:ext[])
                                n220 = Index Array(array=w692, index=w693) -> (element=w691:ext)
                                n221 = global read "musicplayer_glo.vi" "pfade"() -> (w695:string[])
                                n222 = Index Array(array=w695, index=w691) -> (element=w694:string)
                                }
                                }
                              }
                            }
                          }
                        }
                      }
                    }
                    n223 = local write "switch"(FALSE ("switch")) -> ()
                    n224 = global write "musicplayer_glo.vi" "play-alone"(w657) -> ()
                  }
                }
              }
              frame True {
                n225 = case "play alone?" shown="False" w703 {
                  tunnel: [w713 w728] -> w702
                  tunnel: [w711 _] -> w701
                  tunnel: w700 -> [w712 _]
                  tunnel: w699 -> [w710 _]
                  tunnel: [w709 -1] -> w698
                  tunnel: w697 -> [w704 _]
                  frame False {
                    n226 = Not Equal?(x=w704, y=-1.0) -> (x != y?=w705:bool)
                    n227 = Not(x=w705) -> (.not. x?=w706:bool)
                    n228 = And(x=w710, y=w706) -> (x .and. y?=w707:bool)
                    n229 = case "zufall, & kein line-festgelegt?" shown="True" w707 {
                      tunnel: w712 -> [_ w723]
                      tunnel: w704 -> [w717 _]
                      tunnel: [w718 w721] -> w711
                      tunnel: [-1 w722] -> w709
                      tunnel: w705 -> [w716 _]
                      frame False {
                        n230 = case shown="False" w716 {
                          tunnel: [0 w720] -> w718
                          tunnel: w717 -> [_ w720]
                          frame False {
                          }
                          frame True {
                          }
                        }
                      }
                      frame True {
                        n231 = stacked-sequence {
                          tunnel: w723 -> [_ _]
                          tunnel: [_ w726] -> w721
                          tunnel: [_ w725] -> w722
                          frame #0 {
                            n232 = call "write_random_data.vi"() -> ()  [unwired: 12 in]
                          }
                          frame #1 {
                            w725 = 0
                            n233 = global read "musicplayer_glo.vi" "random-data"() -> (w724:ext[])
                            n234 = Index Array(array=w724, index=w725) -> (element=w726:ext)
                          }
                        }
                      }
                    }
                    n235 = global read "musicplayer_glo.vi" "pfade"() -> (w714:string[])
                    n236 = Index Array(array=w714, index=w711) -> (element=w713:string)
                  }
                  frame True {
                    n237 = global read "musicplayer_glo.vi" "playlone-lied-Pfad"() -> (w728:string)
                  }
                }
              }
            }
            n238 = case shown="True" w529 {
              tunnel: w530 -> [_ _]
              tunnel: [2 -1] -> w528
              frame False {
              }
              frame True {
                n239 = global write "musicplayer_glo.vi" "stop-event"(TRUE ("stop-event")) -> ()
              }
            }
            n240 = global write "musicplayer_glo.vi" "play-event"(w520) -> ()
            n241 = String To Path(string=w533) -> (path=w516:path)
            n242 = global write "player_glo.vi" "path"(w516) -> ()
          }
          frame 2 {
            n243 = stacked-sequence {
              tunnel: w733 -> [_ w753]
              tunnel: w732 -> [_ w752]
              tunnel: [_ w746] -> w729
              frame #0 {
                n244 = local read "nachtitelpausieren"() -> (w734:bool)
                n245 = case shown="True" w734 {
                  frame False {
                    (unwired) 3
                  }
                  frame True {
                    n246 = stacked-sequence {
                      frame #0 {
                        w735 = TRUE
                        n247 = local write "pause"(w735) -> ()
                        n248 = local write "pause?"(w735) -> ()
                      }
                      frame #1 {
                        n249 = while {
                          stop <- w741 stop-if-true
                          n250 = Wait Until Next ms Multiple(millisecond multiple=u32 50 ("Vielfache von ms")) -> ()  [unwired: 1 out]
                          n251 = global read "musicplayer_glo.vi" "stop-event"() -> (w738:bool)
                          n252 = global read "musicplayer_glo.vi" "play-event"() -> (w736:bool)
                          n253 = local read "pause?"() -> (w740:bool)
                          n254 = Not(x=w740) -> (.not. x?=w739:bool)
                          n255 = global read "musicplayer_glo.vi" "exit?"() -> (w737:bool)
                          n256 = Compound Arithmetic op=OR(w737, w739, w738, w736) -> (w741:bool)
                        }
                      }
                    }
                  }
                }
              }
              frame #1 {
                # "einzeln abspielen? & play starten, play-buttons deaktivieren ( je nach einzeln oder playlist )"
                n257 = case "play alone?" shown="True" w752 {
                  tunnel: w753 -> [w764 _]
                  tunnel: [T4."Disabled" ("Deaktiviert") T4."Disabled and Grayed Out" ("Deaktiviert")] -> w751
                  tunnel: [T4."Disabled and Grayed Out" ("Deaktiviert") T4."Disabled" ("Deaktiviert")] -> w750
                  frame False {
                    n258 = stacked-sequence {
                      tunnel: w764 -> [w765 _]
                      frame #0 {
                        n259 = global write "musicplayer_glo.vi" "new-line-event-main-line"(w765) -> ()
                      }
                      frame #1 {
                        n260 = global write "musicplayer_glo.vi" "new-line-event-main"(TRUE ("new-line-event-main")) -> ()
                      }
                    }
                  }
                  frame True {
                  }
                }
                n261 = local write "nachtitelpausieren"(FALSE ("nachtitelstoppen")) -> ()
                n262 = global read "musicplayer_glo.vi" "stop-event"() -> (w743:bool)
                n263 = global read "musicplayer_glo.vi" "play-event"() -> (w745:bool)
                n264 = property on="nachtitelpausieren" class="Bool. (strikt)"("DisabledEnum"=T4."Enabled" ("Deaktiviert")) -> ()  [unwired: 2 in, 2 out]
                n265 = global read "musicplayer_glo.vi" "exit?"() -> (w748:bool)
                n266 = Compound Arithmetic op=OR(w745, w748, w743) -> (w747:bool)
                n267 = case shown="True" w747 {
                  tunnel: [3 w758] -> w746
                  tunnel: w745 -> [_ w759]
                  tunnel: w743 -> [_ w756]
                  frame False {
                  }
                  frame True {
                    n268 = Not(x=w756) -> (.not. x?=w755:bool)
                    n269 = And(x=w759, y=w755) -> (x .and. y?=w757:bool)
                    n270 = case "playevent & kein stop ?" shown="False" w757 {
                      tunnel: [-1 1] -> w758
                      frame False {
                        # "nein: resett"
                      }
                      frame True {
                        # "ja: go ahead"
                      }
                    }
                  }
                }
                n271 = property on="play" class="Bool."("DisabledEnum"=w751) -> ()  [unwired: 2 in, 2 out]
                n272 = property on="abspielen-einzeln" class="Bool."("DisabledEnum"=w750) -> ()  [unwired: 2 in, 2 out]
              }
            }
          }
          frame 3 {
            n273 = stacked-sequence {
              tunnel: [_ w782 _] -> w772
              tunnel: [_ w781 _] -> w770
              tunnel: w769 -> [_ _ _]
              frame #0 {
                n274 = global read "player_glo.vi" "path"() -> (w774:path)
                n275 = global write "musicplayer_glo.vi" "playing?"(TRUE ("playing?")) -> ()
                n276 = call <vilib>:"Get File Extension.vi"("file"=w774) -> ("filename without extension"=w775:string)  [unwired: 7 in, 3 out]
                n277 = global write "musicplayer_glo.vi" "titelname"(w775) -> ()
                "pause?" <- FALSE ("pause")
              }
              frame #1 {
                n278 = flat-sequence {
                  tunnel: [w788] -> w780
                  tunnel: [w787] -> w778
                  tunnel: [w811] -> w782
                  tunnel: [w810] -> w781
                  tunnel: w780 -> [w809]
                  tunnel: [TRUE] -> w779
                  tunnel: w778 -> [w806]
                  frame #0 {
                    w784 = 6 items=["wmppsUndefined", "wmppsStopped", "wmppsPaused", "wmppsPlaying", "wmppsScanForward", "wmppsScanReverse", "wmppsBuffering", "wmppsWaiting", "wmppsMediaEnded", "wmppsTransitioning", "wmppsReady", "wmppsReconnecting", "wmppsLast"] ("playState")
                    # "zurücksetzen,\ngrund für notwendigkeit\nunbekannt"
                    n279 = global write "player_glo.vi" "play"(TRUE) -> ()
                    n280 = global write "player_glo.vi" "playState"(w784) -> ()
                  }
                  frame #1 {
                    n281 = disable-structure shown="Deaktiviert" {
                      frame Disabled {
                        # "temp"
                        n282 = Wait (ms)(milliseconds to wait=u32 1000 ("Zu wartende ms")) -> ()  [unwired: 1 out]
                      }
                      frame Enabled {
                      }
                    }
                  }
                  frame #2 {
                    n283 = while {
                      tunnel: [w795] -> w788
                      shift-right: [FALSE] -> _
                      shift-left: TRUE -> [w790]
                      stop <- w794 stop-if-true
                      # "warten auf spieler spielt ab / error & 1 sek. vorbei, um signaloverride zu verhindern"
                      n284 = Wait Until Next ms Multiple(millisecond multiple=u32 50 ("Vielfache von ms")) -> ()  [unwired: 1 out]
                      n285 = global read "player_glo.vi" "zeitmax"() -> (w795:dbl)
                      n286 = call "Verstrichene Zeit"("Reset"=w790, "Auto Reset"=FALSE) -> ("Time has Elapsed"=w792:bool)  [unwired: 10 in, 7 out]
                      n287 = property on="position" class="Schieber (strikt)"("Scale.Maximum"=w795) -> ()  [unwired: 2 in, 2 out]
                      n288 = case shown="True" w792 {
                        selector: w792 -> [w796 _]
                        tunnel: [w796 w802] -> w794
                        frame False {
                        }
                        frame True {
                          w800 = 6 items=["wmppsUndefined", "wmppsStopped", "wmppsPaused", "wmppsPlaying", "wmppsScanForward", "wmppsScanReverse", "wmppsBuffering", "wmppsWaiting", "wmppsMediaEnded", "wmppsTransitioning", "wmppsReady", "wmppsReconnecting", "wmppsLast"] ("playState")
                          w801 = 3 items=["wmppsUndefined", "wmppsStopped", "wmppsPaused", "wmppsPlaying", "wmppsScanForward", "wmppsScanReverse", "wmppsBuffering", "wmppsWaiting", "wmppsMediaEnded", "wmppsTransitioning", "wmppsReady", "wmppsReconnecting", "wmppsLast"] ("playState")
                          n289 = global read "musicplayer_glo.vi" "play-event"() -> (w805:bool)
                          n290 = global read "musicplayer_glo.vi" "stop-event"() -> (w803:bool)
                          n291 = global read "player_glo.vi" "playState"() -> (w799:i32)
                          n292 = Equal?(x=w799, y=w800) -> (x = y?=w798:bool)
                          n293 = Equal?(x=w799, y=w801) -> (x = y?=w797:bool)
                          n294 = global read "player_glo.vi" "error"() -> (w804:bool)
                          n295 = Compound Arithmetic op=OR(w805, w804, w803, w798, w797) -> (w802:bool)
                        }
                      }
                    }
                    n296 = control-ref of="NotifyIcon reference out"() -> (w787:refnum<vi>)
                  }
                  frame #3 {
                    n297 = call "formattitel&showannotation.vi"("reference"=w806) -> ()
                    n298 = while {
                      shift-right: [w827] -> _
                      shift-left: FALSE -> [w828]
                      shift-right: [w822] -> _
                      shift-left: w809 -> [w817]
                      tunnel: [w830] -> w812
                      stop <- w832 stop-if-true
                      w820 = 1 items=["wmppsUndefined", "wmppsStopped", "wmppsPaused", "wmppsPlaying", "wmppsScanForward", "wmppsScanReverse", "wmppsBuffering", "wmppsWaiting", "wmppsMediaEnded", "wmppsTransitioning", "wmppsReady", "wmppsReconnecting", "wmppsLast"] ("playState")
                      # "warten auf titel ende/player stopped/play-event/kernel-error\nschreiben von Balance & Volume"
                      n299 = global read "player_glo.vi" "zeit"() -> (w819:dbl)
                      n300 = global read "musicplayer_glo.vi" "stop-event"() -> (w831:bool)
                      n301 = global read "musicplayer_glo.vi" "play-event"() -> (w829:bool)
                      n302 = Wait Until Next ms Multiple(millisecond multiple=u32 50 ("Vielfache von ms")) -> ()  [unwired: 1 out]
                      n303 = global read "player_glo.vi" "playState"() -> (w821:i32)
                      n304 = global read "player_glo.vi" "zeitmax"() -> (w818:dbl)
                      n305 = local read "pause?"() -> (w826:bool)
                      n306 = local read "playwhile-brake"() -> (w825:bool)
                      n307 = local write "position"(w819) -> ()
                      n308 = Not Equal?(x=w817, y=w818) -> (x != y?=w823:bool)
                      n309 = case shown="False" w828 {
                        selector: w828 -> [w839 w847]
                        tunnel: [w838 w848] -> w827
                        tunnel: w826 -> [w837 w849]
                        tunnel: w821 -> [w836 w846]
                        frame False {
                          n310 = case shown="True" w837 {
                            selector: w837 -> [_ w844]
                            tunnel: w839 -> [w840 _]
                            tunnel: [w840 w844] -> w838
                            tunnel: w836 -> [_ w841]
                            frame False {
                            }
                            frame True {
                              w843 = 3 items=["wmppsUndefined", "wmppsStopped", "wmppsPaused", "wmppsPlaying", "wmppsScanForward", "wmppsScanReverse", "wmppsBuffering", "wmppsWaiting", "wmppsMediaEnded", "wmppsTransitioning", "wmppsReady", "wmppsReconnecting", "wmppsLast"] ("playState")
                              n311 = local write "pause"(w844) -> ()
                              n312 = Equal?(x=w841, y=w843) -> (x = y?=w842:bool)
                              n313 = case shown="True" w842 {
                                frame False {
                                }
                                frame True {
                                n314 = global write "player_glo.vi" "pause"(TRUE) -> ()
                                }
                              }
                            }
                          }
                        }
                        frame True {
                          n315 = case shown="False" w849 {
                            selector: w849 -> [w853 _]
                            tunnel: [w853 w855] -> w848
                            tunnel: w847 -> [_ w855]
                            tunnel: w846 -> [w850 _]
                            frame False {
                              w851 = 2 items=["wmppsUndefined", "wmppsStopped", "wmppsPaused", "wmppsPlaying", "wmppsScanForward", "wmppsScanReverse", "wmppsBuffering", "wmppsWaiting", "wmppsMediaEnded", "wmppsTransitioning", "wmppsReady", "wmppsReconnecting", "wmppsLast"] ("playState")
                              n316 = local write "pause"(w853) -> ()
                              n317 = Equal?(x=w850, y=w851) -> (x = y?=w852:bool)
                              n318 = case shown="False" w852 {
                                frame False {
                                }
                                frame True {
                                n319 = global write "player_glo.vi" "pause"(TRUE) -> ()
                                }
                              }
                            }
                            frame True {
                            }
                          }
                        }
                      }
                      n320 = Compound Arithmetic op=OR "Mehrfacharithmetik"(w831) -> (w830:bool)
                      n321 = case shown="False" w823 {
                        tunnel: w818 -> [_ w835]
                        tunnel: [w834 w835] -> w822
                        tunnel: w817 -> [w834 _]
                        frame False {
                        }
                        frame True {
                          n322 = property on="position" class="Schieber (strikt)"("Scale.Maximum"=w835) -> ()  [unwired: 2 in, 2 out]
                        }
                      }
                      n323 = Equal?(x=w821, y=w820) -> (x = y?=w816:bool)
                      n324 = global read "player_glo.vi" "error"() -> (w824:bool)
                      n325 = Compound Arithmetic op=OR(w825, w829, w816, w831, w824) -> (w832:bool)
                    }
                    n326 = case shown="False" w812 {
                      tunnel: [1 -1] -> w811
                      tunnel: [TRUE _] -> w810
                      frame False {
                      }
                      frame True {
                      }
                    }
                  }
                }
                n327 = global write "player_glo.vi" "stop"(w779) -> ()
              }
              frame #2 {
                w856 = FALSE ("playing?")
                n328 = global write "player_glo.vi" "error"(w856) -> ()
                n329 = global write "musicplayer_glo.vi" "playing?"(w856) -> ()
              }
            }
          }
        }
        n330 = Wait Until Next ms Multiple(millisecond multiple=u32 50 ("Vielfache von ms")) -> ()  [unwired: 1 out]
        n331 = global read "musicplayer_glo.vi" "exit?"() -> (w487:bool)
      }
      n332 = while {
        tunnel: w209 -> [w229]
        shift-right: [w227] -> _
        shift-left: 0 -> [w228]
        shift-right: [w223] -> _
        shift-left: w197 -> [w224]
        tunnel: w193 -> [w220]
        tunnel: w196 -> [w221]
        shift-right: [w218] -> _
        shift-left: w195 -> [w219]
        stop <- w222 stop-if-true
        # "aktualisierungs-dämon"
        n333 = Wait Until Next ms Multiple(millisecond multiple=u32 100 ("Vielfache von ms")) -> ()  [unwired: 1 out]
        n334 = global read "musicplayer_glo.vi" "playing?"() -> (w230:bool)
        n335 = global read "musicplayer_glo.vi" "main-geschlossen?"() -> (w225:bool)
        n336 = global read "musicplayer_glo.vi" "foreground?"() -> (w226:bool)
        n337 = case shown="True" w230 {
          tunnel: [w266 w274] -> w231
          tunnel: w229 -> [w266 _]
          frame False {
          }
          frame True {
            n338 = global write "player_glo.vi" "volume"("Volume") -> ()
            n339 = global read "player_glo.vi" "time-string"() -> (w267:string)
            n340 = global read "musicplayer_glo.vi" "titelname"() -> (w272:string)
            n341 = local read "pause?"() -> (w273:bool)
            n342 = Multiply(x=i8 10, y="balance") -> (x*y=w270:i8)
            n343 = global write "player_glo.vi" "balance"(w270) -> ()
            n344 = call "Titelsteuerung.vi"("time-string"=w267, "titel"=w272, "Pause"=w273) -> ("String"=w274:string)  [unwired: 1 in]
          }
        }
        n345 = case "sichtbarkeits-handler" shown="0, Standard" w224 {
          selector: w224 -> [w235 w243]
          tunnel: w225 -> [w236 w245]
          tunnel: [w234 w244] -> w223
          tunnel: w220 -> [w233 w242]
          frame 0, Default {
            n346 = case shown="False" w236 {
              tunnel: w235 -> [w237 w239]
              tunnel: [w237 w238] -> w234
              tunnel: w233 -> [_ w241]
              frame False {
              }
              frame True {
                n347 = Increment(x=w239) -> (x+1=w238:i32)
                n348 = property class="VI"(reference=w241, "FP.State"=T2."Hidden" ("Frontpanel-Fenster:Status")) -> ()  [unwired: 1 in, 2 out]
              }
            }
          }
          frame 1 {
            n349 = case shown="True" w245 {
              tunnel: [0 w249] -> w244
              tunnel: w243 -> [_ w249]
              tunnel: w242 -> [w246 _]
              frame False {
                n350 = property class="VI"(reference=w246, "FP.State"=T2."Standard" ("Frontpanel-Fenster:Status")) -> ()  [unwired: 1 in, 2 out]
              }
              frame True {
              }
            }
          }
        }
        n351 = case shown="False" w226 {
          tunnel: w228 -> [w252 _]
          tunnel: [w250 _] -> w227
          tunnel: w221 -> [w251 w260]
          tunnel: w219 -> [_ w259]
          tunnel: [_ w258] -> w218
          frame False {
            n352 = case shown="0, Standard" w252 {
              selector: w252 -> [w255 w257]
              tunnel: [w256 w257] -> w250
              tunnel: w251 -> [w254 _]
              frame 0, Default {
                n353 = Increment(x=w255) -> (x+1=w256:i32)
                n354 = call "Revoke Window Always on Top.vi"("activate? (F)"=TRUE, "window refnum (NaWR)"=w254) -> ()  [unwired: 4 in, 2 out]
              }
              frame 1 {
              }
            }
          }
          frame True {
            n355 = case shown="1" w259 {
              selector: w259 -> [w263 w265]
              tunnel: w260 -> [w264 _]
              tunnel: [w262 w265] -> w258
              frame 0, Default {
                n356 = Increment(x=w263) -> (x+1=w262:i32)
                n357 = call "Make Window Always on Top.vi"("activate? (F)"=TRUE, "window refnum (NaWR)"=w264) -> ()  [unwired: 4 in, 2 out]
              }
              frame 1 {
              }
            }
          }
        }
        n358 = property class="VI"(reference=w220, "Front Panel.Title"=w231) -> ()  [unwired: 1 in, 2 out]
        n359 = global read "musicplayer_glo.vi" "exit?"() -> (w222:bool)
      }
      n360 = call "NotifyIcon - Register LabVIEW User Events.vi"("Action"=NotifyIcon_Event_Registration_Actions."Initial Event Registration", "Events to register"=w206, "NotifyIcon reference in"=w207) -> ("Event Registration Refnum"=w202:refnum<event-registration>, "NotifyIcon reference out"=→"NotifyIcon reference out":refnum<k24>)  [unwired: 6 in, 1 out]
      n361 = while {
        tunnel: w193 -> [w278]
        tunnel: w211 -> [w283]
        tunnel: w202 -> [w282]
        tunnel: w200 -> [w281]
        tunnel: w199 -> [w280]
        tunnel: w198 -> [w279]
        tunnel: [w276] -> w194
        stop <- w277 stop-if-true
        n362 = global read "musicplayer_glo.vi" "deutsch?"() -> (w284:bool)
        n363 = event shown="[1] Menüauswahl (Benutzer)" {
          selector: w282 -> [_ _ _ _ _ _ _ _ _ _ _ _ _]
          dyn-events: [_ _ _ _ _ _ _ _ _ _ _ _ _] -> w276
          timeout: 50 -> [_ _ _ _ _ _ _ _ _ _ _ _ _]
          tunnel: w284 -> [_ w295 w349 _ _ _ _ _ w459 _ _ _ w477]
          tunnel: w283 -> [_ w296 _ _ _ _ _ _ w458 _ _ _ _]
          tunnel: w281 -> [_ w294 _ _ _ _ _ _ _ _ _ _ _]
          tunnel: w280 -> [_ w293 _ _ _ _ _ _ _ _ _ _ _]
          tunnel: w279 -> [_ w292 _ _ _ _ _ _ _ _ _ _ _]
          tunnel: w278 -> [_ _ w348 _ _ _ _ _ _ _ _ _ w476]
          event "play": Value Change {
            n364 = event-data() -> ()  [unwired: 1 in, 5 out]
            n365 = global read "musicplayer_glo.vi" "pfade"() -> (w288:string[])
            n366 = Array Size(array=w288) -> (size(s)=w287:i32)
            n367 = Not Equal?(x=w287, y=0) -> (x != y?=w285:bool)
            n368 = case shown="True" w285 {
              frame False {
              }
              frame True {
                n369 = stacked-sequence {
                  frame #0 {
                    n370 = global write "musicplayer_glo.vi" "play-alone"(FALSE ("play-alone")) -> ()
                    n371 = global write "musicplayer_glo.vi" "play-event-line"(-1) -> ()
                  }
                  frame #1 {
                    n372 = global write "musicplayer_glo.vi" "play-event"(TRUE ("play-event")) -> ()
                  }
                }
              }
            }
          }
          event Menu Selection (User) {
            n373 = event-data() -> ("ItemTag"=w298:string)  [unwired: 1 in, 5 out]
            n374 = case shown="\"Play_Pause\"" w298 {
              tunnel: [_ TRUE _ _ _ _ _ _ _ _ _ _ _ _ _] -> _
              tunnel: [_ _ _ _ _ _ _ TRUE TRUE FALSE FALSE _ _ _ _] -> w297
              tunnel: w296 -> [_ _ _ _ _ _ _ _ _ _ _ w338 _ _ _]
              tunnel: w295 -> [_ w300 _ _ _ _ _ _ _ _ _ _ w341 w344 _]
              tunnel: w294 -> [_ _ _ _ _ _ _ _ _ _ _ _ w340 w347 _]
              tunnel: w293 -> [_ _ _ _ _ _ _ _ _ _ _ _ _ w346 _]
              tunnel: w292 -> [_ _ _ _ _ _ _ _ _ _ _ _ _ w345 _]
              frame "default", Default {
              }
              frame "Close" {
                n375 = control-ref of="Volume"() -> (w303:refnum<vi>)
                n376 = control-ref of="balance"() -> (w302:refnum<vi>)
                n377 = control-ref of="verdeckung"() -> (w306:refnum<vi>)
                n378 = control-ref of="Dieses VI"() -> (w301:refnum<vi>)
                n379 = control-ref of="configPfad"() -> (w304:refnum<vi>)
                n380 = control-ref of="NotifyIcon reference out"() -> (w305:refnum<vi>)
                n381 = call "exit_main.vi"("Dieses VI"=w301, "deutsch?"=w300, "balance"=w302, "volume"=w303, "configPfad"=w304, "notifyicon_reference"=w305, "verdeckung"=w306) -> ()  [unwired: 1 in]
              }
              frame "Show" {
                n382 = global write "musicplayer_glo.vi" "playlist sichtbar?"(TRUE ("playlist sichtbar?")) -> ()
                n383 = local read "playlist referenz"() -> (w312:refnum<vi>)
                n384 = property class="VI"(reference=w312) -> (reference out=w308:refnum<vi>, "FP.State"=w311:T2)  [unwired: 1 in, 1 out]
                n385 = Equal?(x=w311, y=T2."Minimized") -> (x = y?=w309:bool)
                n386 = case shown="False" w309 {
                  tunnel: w308 -> [_ w315]
                  frame False {
                  }
                  frame True {
                    n387 = property class="VI"(reference=w315, "FP.State"=T2."Standard" ("Frontpanel-Fenster:Status")) -> ()  [unwired: 1 in, 2 out]
                  }
                }
              }
              frame "Clear Playlist" {
                n388 = call "Meldung an Benutzer8"("Message"="Sorry.\nThis function if comming soon.\nPlease do rightklick on the Playlist for this function.") -> ()  [unwired: 9 in, 2 out]
              }
              frame "Play_Pause" {
                n389 = global read "musicplayer_glo.vi" "playing?"() -> (w317:bool)
                n390 = case shown="True" w317 {
                  frame False {
                    n391 = global read "musicplayer_glo.vi" "pfade"() -> (w321:string[])
                    n392 = Array Size(array=w321) -> (size(s)=w320:i32)
                    n393 = Not Equal?(x=w320, y=0) -> (x != y?=w318:bool)
                    n394 = case shown="True" w318 {
                      frame False {
                      }
                      frame True {
                        n395 = stacked-sequence {
                          frame #0 {
                            n396 = global write "musicplayer_glo.vi" "play-alone"(FALSE ("play-alone")) -> ()
                            n397 = global write "musicplayer_glo.vi" "play-event-line"(-1) -> ()
                          }
                          frame #1 {
                            n398 = global write "musicplayer_glo.vi" "play-event"(TRUE ("play-event")) -> ()
                          }
                        }
                      }
                    }
                  }
                  frame True {
                    n399 = local read "pause?"() -> (w326:bool)
                    n400 = Not(x=w326) -> (.not. x?=w325:bool)
                    n401 = local write "pause?"(w325) -> ()
                  }
                }
              }
              frame "Ever in foreground" {
                n402 = global read "musicplayer_glo.vi" "foreground?"() -> (w328:bool)
                n403 = Not(x=w328) -> (.not. x?=w327:bool)
                n404 = global write "musicplayer_glo.vi" "foreground?"(w327) -> ()
              }
              frame "Titel-Info" {
                n405 = global read "musicplayer_glo.vi" "titel-info?"() -> (w330:bool)
                n406 = Not(x=w330) -> (.not. x?=w329:bool)
                n407 = global write "musicplayer_glo.vi" "titel-info?"(w329) -> ()
              }
              frame "Lock Musicplayer" {
              }
              frame "Help_1" {
              }
              frame "Load Playlist" {
                n408 = call "Meldung an Benutzer5"("Message"="Sorry.\nThis function if comming soon.\nPlease do rightklick on the Playlist for this function.") -> ()  [unwired: 9 in, 2 out]
              }
              frame "Save Playlist" {
                n409 = call "Meldung an Benutzer6"("Message"="Sorry.\nThis function if comming soon.\nPlease do rightklick on the Playlist for this function.") -> ()  [unwired: 9 in, 2 out]
              }
              frame "Filetypes" {
                n410 = Concatenate Strings("This Programm is using a part of Microsoft kernel (c)\nVideos are support too, but are playing without picture.\nSome Videos with a different kb/s does make errors.\nThis error does not come from this Software, and is from\nMicrosoft.\nSupported files:\n", w338) -> (w337:string)
                n411 = call "Meldung an Benutzer7"("Message"=w337) -> ()  [unwired: 9 in, 2 out]
              }
              frame "About" {
                n412 = call "Info.vi"("deutsch?"=w341, "virsualisierung?"=FALSE, "Version"=w340) -> ()  [unwired: 9 in]
              }
              frame "Check for updates" {
                n413 = call "check_updates.vi"("dialog by newest version?"=TRUE, "german?"=w344, "downloadpath"=w346, "get-path"=w345, "current version"=w347) -> ()  [unwired: 6 in, 1 out]
              }
              frame "Debug" {
              }
            }
            n414 = case shown="True" w297 {
              frame False {
              }
              frame True {
                n415 = call "Meldung an Benutzer4"("Message"="Sorry.\nThis function is comming soon." ("String")) -> ()  [unwired: 9 in, 2 out]
              }
            }
          }
          event User Event {
            # "task-icon-event-handler"
            n416 = event-data() -> ("Event Data"=w355:variant)  [unwired: 1 in, 3 out]
            n417 = call "NotifyIcon - Interpret Event Data.vi"("NotifyIcon Event Data"=w355) -> ("error out"=w351:errorcluster, "NotifyIcon Event Data"=w354:T7)  [unwired: 9 in]
            n418 = Unbundle By Name(w354) -> ("NotifyIcon Event"=w353:T6, "Data String"=w352:string)
            n419 = case shown="\"MenuItemSelect\"" w353 {
              tunnel: w352 -> [_ _ _ _ _ _ _ _ _ _ _ w412 _]
              tunnel: w351 -> [_ w370 _ _ _ _ _ _ _ _ _ _ _]
              tunnel: [_ w369 _ _ _ _ _ _ _ _ _ _ _] -> _
              tunnel: [_ _ _ _ _ _ _ _ _ _ _ w410 _] -> w350
              frame "BalloonTipClicked" {
                n420 = stacked-sequence {
                  frame #0 {
                    n421 = control-ref of="Dieses VI"() -> (w365:refnum<vi>)
                    n422 = property class="VI"(reference=w365, "FP.State"=T2."Minimized" ("Frontpanel-Fenster:Status"), "FP:RunTransparently"=TRUE ("Frontpanel-Fenster:VI transparent ausführen")) -> ()  [unwired: 1 in, 2 out]
                  }
                  frame #1 {
                    n423 = control-ref of="Dieses VI"() -> (w368:refnum<vi>)
                    n424 = property class="VI"(reference=w368, "FP.State"=T2."Standard" ("Frontpanel-Fenster:Status"), "FP:RunTransparently"=TRUE ("Frontpanel-Fenster:VI transparent ausführen")) -> ()  [unwired: 1 in, 2 out]
                  }
                }
              }
              frame "BalloonTipClosed", Default {
                # "imprinzip default"
                n425 = call <vilib>:"Error Cluster From Error Code.vi"("error in (no error)"=w370, "error message (\"\")"="NotifyIcon event not handled." ("error message (\"\")"), "error code (0)"=7000) -> ("error out"=w369:errorcluster)  [unwired: 6 in]
              }
              frame "BalloonTipShown" {
              }
              frame "Click" {
              }
              frame "Disposed" {
              }
              frame "DoubleClick" {
                # "show/hide musicplayer"
                n426 = control-ref of="Dieses VI"() -> (w385:refnum<vi>)
                n427 = local read "playlist referenz"() -> (w380:refnum<vi>)
                n428 = property class="VI"(reference=w385) -> (reference out=w382:refnum<vi>, "FP.State"=w383:T2)  [unwired: 1 in, 1 out]
                n429 = property class="VI"(reference=w380) -> (reference out=w379:refnum<vi>, "FP.State"=w376:T2)  [unwired: 1 in, 1 out]
                n430 = Not Equal?(x=w376, y=T2."Hidden") -> (x != y?=w373:bool)
                n431 = Equal?(x=w376, y=T2."Minimized") -> (x = y?=w378:bool)
                n432 = Equal?(x=w383, y=T2."Minimized") -> (x = y?=w374:bool)
                n433 = case shown="False" w374 {
                  tunnel: w382 -> [w400 w401]
                  frame False {
                    n434 = property class="VI"(reference=w400, "FP.State"=T2."Minimized" ("Frontpanel-Fenster:Status")) -> ()  [unwired: 1 in, 2 out]
                  }
                  frame True {
                    n435 = stacked-sequence {
                      tunnel: w401 -> [w402 w405]
                      frame #0 {
                        n436 = property class="VI"(reference=w402, "FP.State"=T2."Minimized" ("Frontpanel-Fenster:Status"), "FP:RunTransparently"=TRUE ("Frontpanel-Fenster:VI transparent ausführen")) -> ()  [unwired: 1 in, 2 out]
                      }
                      frame #1 {
                        n437 = property class="VI"(reference=w405, "FP.State"=T2."Standard" ("Frontpanel-Fenster:Status"), "FP:RunTransparently"=TRUE ("Frontpanel-Fenster:VI transparent ausführen")) -> ()  [unwired: 1 in, 2 out]
                      }
                    }
                  }
                }
                n438 = Compound Arithmetic op=OR(w378, w374) -> (w377:bool)
                n439 = case shown="True" w377 {
                  tunnel: w379 -> [w387 w391]
                  tunnel: w373 -> [w386 w390]
                  frame False {
                    n440 = case shown="True" w386 {
                      tunnel: w387 -> [_ w388]
                      frame False {
                      }
                      frame True {
                        n441 = property class="VI"(reference=w388, "FP.State"=T2."Minimized" ("Frontpanel-Fenster:Status")) -> ()  [unwired: 1 in, 2 out]
                      }
                    }
                  }
                  frame True {
                    n442 = case shown="True" w390 {
                      tunnel: w391 -> [_ w392]
                      frame False {
                      }
                      frame True {
                        n443 = stacked-sequence {
                          tunnel: w392 -> [w393 w396]
                          frame #0 {
                            n444 = property class="VI"(reference=w393, "FP.State"=T2."Minimized" ("Frontpanel-Fenster:Status"), "FP:RunTransparently"=TRUE ("Frontpanel-Fenster:VI transparent ausführen")) -> ()  [unwired: 1 in, 2 out]
                          }
                          frame #1 {
                            n445 = property class="VI"(reference=w396, "FP.State"=T2."Standard" ("Frontpanel-Fenster:Status"), "FP:RunTransparently"=TRUE ("Frontpanel-Fenster:VI transparent ausführen")) -> ()  [unwired: 1 in, 2 out]
                          }
                        }
                      }
                    }
                  }
                }
              }
              frame "MouseClick" {
              }
              frame "MouseDoubleClick" {
              }
              frame "MouseDown" {
              }
              frame "MouseMove" {
              }
              frame "MouseUp" {
                n446 = local read "Volume"() -> (w408:i64)
                n447 = Increment(x=w408) -> (x+1=w409:i64)
                n448 = local write "Volume"(w409) -> ()
              }
              frame "MenuItemClick" {
                # "menu-clicked"
                n449 = Match Pattern(string=w412, regular expression="\\" ("Regulärer Ausdruck")) -> (after substring=w413:string, offset past match=w414:i32)  [unwired: 1 in, 2 out]
                n450 = Equal?(x=w414, y=-1) -> (x = y?=w416:bool)
                n451 = case shown="True" w416 {
                  tunnel: w413 -> [w439 _]
                  tunnel: [w439 w440] -> w411
                  tunnel: w412 -> [_ w440]
                  frame False {
                  }
                  frame True {
                  }
                }
                n452 = case shown="\"Stop\"" w411 {
                  tunnel: [_ _ TRUE _ _ _] -> w410
                  frame "default", Default {
                    # "default-case"
                  }
                  frame "Stop" {
                    n453 = global write "musicplayer_glo.vi" "stop-event"(TRUE ("stop-event")) -> ()
                  }
                  frame "Beenden", "Exit" {
                  }
                  frame "Play-Pause" {
                    n454 = global read "musicplayer_glo.vi" "playing?"() -> (w422:bool)
                    n455 = local read "nachtitelpausieren"() -> (w420:bool)
                    n456 = Or(x=w420, y=w422) -> (x .or. y?=w421:bool)
                    n457 = case shown="True" w421 {
                      frame False {
                        n458 = global read "musicplayer_glo.vi" "pfade"() -> (w426:string[])
                        n459 = Array Size(array=w426) -> (size(s)=w425:i32)
                        n460 = Not Equal?(x=w425, y=0) -> (x != y?=w423:bool)
                        n461 = case shown="True" w423 {
                          frame False {
                          }
                          frame True {
                            n462 = stacked-sequence {
                              frame #0 {
                                n463 = global write "musicplayer_glo.vi" "play-alone"(FALSE ("play-alone")) -> ()
                                n464 = global write "musicplayer_glo.vi" "play-event-line"(-1) -> ()
                              }
                              frame #1 {
                                n465 = global write "musicplayer_glo.vi" "play-event"(TRUE ("play-event")) -> ()
                              }
                            }
                          }
                        }
                      }
                      frame True {
                        n466 = local read "pause?"() -> (w431:bool)
                        n467 = Not(x=w431) -> (.not. x?=w430:bool)
                        n468 = local write "pause?"(w430) -> ()
                      }
                    }
                  }
                  frame "Musicplayer Öffnen", "Open Musicplayer" {
                    n469 = stacked-sequence {
                      frame #0 {
                        n470 = control-ref of="Dieses VI"() -> (w434:refnum<vi>)
                        n471 = property class="VI"(reference=w434, "FP.State"=T2."Minimized" ("Frontpanel-Fenster:Status"), "FP:RunTransparently"=TRUE ("Frontpanel-Fenster:VI transparent ausführen")) -> ()  [unwired: 1 in, 2 out]
                      }
                      frame #1 {
                        n472 = control-ref of="Dieses VI"() -> (w437:refnum<vi>)
                        n473 = property class="VI"(reference=w437, "FP.State"=T2."Standard" ("Frontpanel-Fenster:Status"), "FP:RunTransparently"=TRUE ("Frontpanel-Fenster:VI transparent ausführen")) -> ()  [unwired: 1 in, 2 out]
                      }
                    }
                  }
                  frame "Next Titel", "Nächsten Titel" {
                    # "Nächsten Titel"
                    n474 = local write "playwhile-brake"(TRUE ("playwhile-brake")) -> ()
                  }
                }
              }
              frame "MenuItemSelect" {
              }
            }
            n475 = case shown="True" w350 {
              tunnel: w349 -> [_ w362]
              tunnel: w348 -> [_ w361]
              frame False {
              }
              frame True {
                n476 = control-ref of="Volume"() -> (w359:refnum<vi>)
                n477 = control-ref of="balance"() -> (w360:refnum<vi>)
                n478 = control-ref of="verdeckung"() -> (w357:refnum<vi>)
                n479 = control-ref of="configPfad"() -> (w358:refnum<vi>)
                n480 = control-ref of="NotifyIcon reference out"() -> (w356:refnum<vi>)
                n481 = call "exit_main.vi"("Dieses VI"=w361, "deutsch?"=w362, "balance"=w360, "volume"=w359, "configPfad"=w358, "notifyicon_reference"=w356, "verdeckung"=w357) -> ()  [unwired: 1 in]
              }
            }
          }
          event Timeout {
            n482 = event-data() -> ()  [unwired: 1 in, 2 out]
          }
          event "nechstentitel": Value Change {
            n483 = event-data() -> ("NewVal"=w441:bool)  [unwired: 1 in, 4 out]
            n484 = case shown="True" w441 {
              frame False {
              }
              frame True {
                n485 = local write "playwhile-brake"(TRUE) -> ()
              }
            }
          }
          event "pause": Value Change {
            n486 = event-data() -> ()  [unwired: 1 in, 5 out]
            n487 = global read "musicplayer_glo.vi" "playing?"() -> (w445:bool)
            n488 = local read "nachtitelpausieren"() -> (w443:bool)
            n489 = Or(x=w445, y=w443) -> (x .or. y?=w444:bool)
            n490 = case shown="True" w444 {
              frame False {
              }
              frame True {
                n491 = local read "pause?"() -> (w447:bool)
                n492 = Not(x=w447) -> (.not. x?=w446:bool)
                n493 = local write "pause?"(w446) -> ()
              }
            }
          }
          event "position": Value Change {
            n494 = event-data() -> ("NewVal"=w449:ext)  [unwired: 1 in, 4 out]
            n495 = global read "musicplayer_glo.vi" "playing?"() -> (w448:bool)
            n496 = case shown="True" w448 {
              tunnel: w449 -> [_ w450]
              frame False {
              }
              frame True {
                n497 = stacked-sequence {
                  tunnel: w450 -> [w451 _]
                  frame #0 {
                    n498 = global write "player_glo.vi" "set-zeit"(w451) -> ()
                  }
                  frame #1 {
                    n499 = global write "player_glo.vi" "set zeit"(TRUE ("positions änderung")) -> ()
                  }
                }
              }
            }
          }
          event "abspielen-einzeln": Value Change {
            n500 = event-data() -> ()  [unwired: 1 in, 5 out]
            n501 = global read "musicplayer_glo.vi" "playlone-lied-Pfad"() -> (w455:string)
            n502 = Not Equal?(x=w455, y="") -> (x != y?=w453:bool)
            n503 = case shown="True" w453 {
              frame False {
              }
              frame True {
                n504 = stacked-sequence {
                  frame #0 {
                    n505 = global write "musicplayer_glo.vi" "play-alone"(TRUE ("play-alone")) -> ()
                  }
                  frame #1 {
                    n506 = global write "musicplayer_glo.vi" "play-event"(TRUE ("play-event")) -> ()
                  }
                }
              }
            }
          }
          event "playalone-titel": Shortcut Menu Selection (User) {
            n507 = event-data() -> ("ItemTag"=w460:string)  [unwired: 1 in, 6 out]
            n508 = case shown="\"default\", Standard" w460 {
              tunnel: w459 -> [w467 _]
              tunnel: w458 -> [w466 _]
              frame "CHOOSE_TITEL" {
                n509 = global read "musicplayer_glo.vi" "playlone-lied-Pfad"() -> (w465:string)
                n510 = String To Path(string=w465) -> (path=w464:path)
                n511 = call "choose_single.vi"("filetypes"=w466, "Pfad in"=w464, "deutsch?"=w467) -> ("Pfad out"=w462:path)  [unwired: 8 in]
                n512 = Path To String(path=w462) -> (string=w463:string)
                n513 = call <vilib>:"Get File Extension.vi"("file"=w462) -> ("filename without extension"=w461:string)  [unwired: 7 in, 3 out]
                n514 = global write "musicplayer_glo.vi" "playlone-lied-Pfad"(w463) -> ()
                n515 = local write "playalone-titel"(w461) -> ()
              }
              frame "default", Default {
              }
            }
          }
          event Menu Activation? {
            n516 = event-data() -> ("MenuRef"=w471:refnum<k9>)  [unwired: 1 in, 3 out]
            n517 = global read "musicplayer_glo.vi" "titel-info?"() -> (w468:bool)
            n518 = global read "musicplayer_glo.vi" "foreground?"() -> (w472:bool)
            n519 = Set Menu Item Info(6:w472, 7:"Ever in foreground" ("Menüpunkt-Tags"), 11:w471) -> (3:w469:refnum<k9>)  [unwired: 4 in, 1 out]
            n520 = Set Menu Item Info(6:w468, 7:"Titel-Info" ("Menüpunkt-Tags"), 11:w469) -> ()  [unwired: 4 in, 2 out]
            n521 = event-data() -> ()  [unwired: 2 in, 1 out]
          }
          event "zufall": Value Change {
            n522 = event-data() -> ("NewVal"=w474:bool)  [unwired: 1 in, 4 out]
            n523 = global write "musicplayer_glo.vi" "random?"(w474) -> ()
          }
          event "stop": Value Change {
            n524 = event-data() -> ()  [unwired: 1 in, 5 out]
            n525 = global write "musicplayer_glo.vi" "stop-event"(TRUE ("stop-event")) -> ()
          }
          event Panel Close? {
            n526 = event-data() -> ()  [unwired: 1 in, 3 out]
            n527 = control-ref of="Volume"() -> (w481:refnum<vi>)
            n528 = control-ref of="balance"() -> (w482:refnum<vi>)
            n529 = control-ref of="verdeckung"() -> (w478:refnum<vi>)
            n530 = control-ref of="configPfad"() -> (w480:refnum<vi>)
            n531 = control-ref of="NotifyIcon reference out"() -> (w479:refnum<vi>)
            n532 = call "exit_main.vi"("Dieses VI"=w476, "deutsch?"=w477, "balance"=w482, "volume"=w481, "configPfad"=w480, "notifyicon_reference"=w479, "verdeckung"=w478) -> ()  [unwired: 1 in]
            n533 = event-data("Discard?"=TRUE ("Verwerfen?")) -> ()  [unwired: 1 in, 1 out]
          }
        }
        n534 = global read "musicplayer_glo.vi" "exit?"() -> (w277:bool)
      }
      n535 = Unregister For Events(event registration refnum=w194) -> ()  [unwired: 1 in, 1 out]
    }
    frame #4 {
      n536 = invoke class="VI" method="FP.Schließen"(reference=w857) -> ()  [unwired: 2 in, 3 out]
    }
  }
